vi "RLmodel GNSS-NtripClient.vi"() -> ()   [LabVIEW 2019]
uses:
  C:/Users/WEGO/Documents/GitHub/Ycar/LabVIEW/Gmap/dll/GMap.NET.WindowsForms.dll
  Gmap/dll/GMap.NET.WindowsForms.dll
  Ctrl/ublox-ui_main.ctl
  Ctrl/gnss_config-2.ctl
  Ctrl/Ntrip_Account_db.ctl
  Ctrl/cmd_common.ctl
  Ctrl/cmd_ini-add-read.ctl
  Ctrl/cmd_ini-RW.ctl
  Ctrl/GNSS-Ntrip ref.ctl
  Gmap/gmap_fgv-cmd.ctl
panel:
  out "GNSS time":string
  out "Ntrip conn":bool
  out "NMEA val":bool
  in  "main tap":T1(tab)
  in  "Send-Serial Start-Stop":bool
  in  "GNSS Start-Stop":bool
  out "TM\nptn":u32(slide) scale=0.0..200.0
  in  "GMapControl":refnum<k24>(container)
  out "Sea Level":dbl
  out "N of Satellites":i32
  out "TM graph":T2(graph)=[{"TM array"=[{"Y(E)"=195478.83340938148, "X(N)"=532749.6315443226}, {"Y(E)"=195478.83340938148, "X(N)"=532749.6315443226}, {"Y(E)"=195478.83340938148, "X(N)"=532749.6315443226}, {"Y(E)"=195478.83340938148, "X(N)"=532749.6315443226}, {"Y(E)"=195478.83340938148, "X(N)"=532749.6315443226}, {"Y(E)"=195478.83340938148, "X(N)"=532749.6315443226}, {"Y(E)"=195478.83340938148, "X(N)"=532749.6315443226}, {"Y(E)"=195478.83340938148, "X(N)"=532749.6315443226}, {"Y(E)"=195478.83340938148, "X(N)"=532749.6315443226}, {"Y(E)"=195478.83340938148, "X(N)"=532749.6315443226}, {"Y(E)"=195478.80387262133, "X(N)"=532749.5945652778}, {"Y(E)"=195478.80387262133, "X(N)"=532749.5945652778}, {"Y(E)"=195478.80387262133, "X(N)"=532749.5945652778}, {"Y(E)"=195478.80387262133, "X(N)"=532749.5945652778}, {"Y(E)"=195478.80387262133, "X(N)"=532749.5945652778}, {"Y(E)"=195478.80387262133, "X(N)"=532749.5945652778}, {"Y(E)"=195478.80387262133, "X(N)"=532749.5945652778}, {"Y(E)"=195478.80387262133, "X(N)"=532749.5945652778}, {"Y(E)"=195478.80387262133, "X(N)"=532749.5945652778}, {"Y(E)"=195478.80387262133, "X(N)"=532749.5945652778}, {"Y(E)"=195478.80387262133, "X(N)"=532749.5945652778}, {"Y(E)"=195478.80387262133, "X(N)"=532749.5945652778}, {"Y(E)"=195478.80387262133, "X(N)"=532749.5945652778}, {"Y(E)"=195478.86283602339, "X(N)"=532749.4650507653}, {"Y(E)"=195478.86283602339, "X(N)"=532749.4650507653}, {"Y(E)"=195478.86283602339, "X(N)"=532749.4650507653}, {"Y(E)"=195478.86283602339, "X(N)"=532749.4650507653}, {"Y(E)"=195478.86283602339, "X(N)"=532749.4650507653}, {"Y(E)"=195478.86283602339, "X(N)"=532749.4650507653}, {"Y(E)"=195478.86283602339, "X(N)"=532749.4650507653}, {"Y(E)"=195478.86283602339, "X(N)"=532749.4650507653}, {"Y(E)"=195478.86283602339, "X(N)"=532749.4650507653}, {"Y(E)"=195478.86283602339, "X(N)"=532749.4650507653}, {"Y(E)"=195478.86283602339, "X(N)"=532749.4650507653}, {"Y(E)"=195478.86283602339, "X(N)"=532749.4650507653}, {"Y(E)"=195478.86283602339, "X(N)"=532749.4650507653}, {"Y(E)"=195478.8185809412, "X(N)"=532749.5020697443}, {"Y(E)"=195478.8185809412, "X(N)"=532749.5020697443}, {"Y(E)"=195478.8185809412, "X(N)"=532749.5020697443}, {"Y(E)"=195478.8185809412, "X(N)"=532749.5020697443}, {"Y(E)"=195478.8185809412, "X(N)"=532749.5020697443}, {"Y(E)"=195478.8185809412, "X(N)"=532749.5020697443}, {"Y(E)"=195478.8185809412, "X(N)"=532749.5020697443}, {"Y(E)"=195478.8185809412, "X(N)"=532749.5020697443}, {"Y(E)"=195478.8185809412, "X(N)"=532749.5020697443}, {"Y(E)"=195478.8185809412, "X(N)"=532749.5020697443}, {"Y(E)"=195478.8185809412, "X(N)"=532749.5020697443}, {"Y(E)"=195478.8185809412, "X(N)"=532749.5020697443}, {"Y(E)"=195478.8185809412, "X(N)"=532749.5020697443}, {"Y(E)"=195478.8333493192, "X(N)"=532749.5205592669}, {"Y(E)"=195478.8333493192, "X(N)"=532749.5205592669}, {"Y(E)"=195478.8333493192, "X(N)"=532749.5205592669}, {"Y(E)"=195478.8333493192, "X(N)"=532749.5205592669}, {"Y(E)"=195478.8333493192, "X(N)"=532749.5205592669}, {"Y(E)"=195478.8333493192, "X(N)"=532749.5205592669}, {"Y(E)"=195478.8333493192, "X(N)"=532749.5205592669}, {"Y(E)"=195478.8333493192, "X(N)"=532749.5205592669}, {"Y(E)"=195478.8333493192, "X(N)"=532749.5205592669}, {"Y(E)"=195478.8333493192, "X(N)"=532749.5205592669}, {"Y(E)"=195478.8333493192, "X(N)"=532749.5205592669}, {"Y(E)"=195478.8333493192, "X(N)"=532749.5205592669}, {"Y(E)"=195478.81854089958, "X(N)"=532749.4280797082}, {"Y(E)"=195478.81854089958, "X(N)"=532749.4280797082}, {"Y(E)"=195478.81854089958, "X(N)"=532749.4280797082}, {"Y(E)"=195478.81854089958, "X(N)"=532749.4280797082}, {"Y(E)"=195478.81854089958, "X(N)"=532749.4280797082}, {"Y(E)"=195478.81854089958, "X(N)"=532749.4280797082}, {"Y(E)"=195478.81854089958, "X(N)"=532749.4280797082}, {"Y(E)"=195478.81854089958, "X(N)"=532749.4280797082}, {"Y(E)"=195478.81854089958, "X(N)"=532749.4280797082}, {"Y(E)"=195478.81854089958, "X(N)"=532749.4280797082}, {"Y(E)"=195478.81854089958, "X(N)"=532749.4280797082}, {"Y(E)"=195478.81854089958, "X(N)"=532749.4280797082}, {"Y(E)"=195478.81854089958, "X(N)"=532749.4280797082}, {"Y(E)"=195478.8332592258, "X(N)"=532749.3540816847}, {"Y(E)"=195478.8332592258, "X(N)"=532749.3540816847}, {"Y(E)"=195478.8332592258, "X(N)"=532749.3540816847}, {"Y(E)"=195478.8332592258, "X(N)"=532749.3540816847}, {"Y(E)"=195478.8332592258, "X(N)"=532749.3540816847}, {"Y(E)"=195478.8332592258, "X(N)"=532749.3540816847}, {"Y(E)"=195478.8332592258, "X(N)"=532749.3540816847}, {"Y(E)"=195478.8332592258, "X(N)"=532749.3540816847}, {"Y(E)"=195478.8332592258, "X(N)"=532749.3540816847}, {"Y(E)"=195478.8332592258, "X(N)"=532749.3540816847}, {"Y(E)"=195478.8332592258, "X(N)"=532749.3540816847}, {"Y(E)"=195478.8332592258, "X(N)"=532749.3540816847}, {"Y(E)"=195478.8332592258, "X(N)"=532749.3540816847}, {"Y(E)"=195478.61200383154, "X(N)"=532749.5761715989}, {"Y(E)"=195478.61200383154, "X(N)"=532749.5761715989}, {"Y(E)"=195478.61200383154, "X(N)"=532749.5761715989}, {"Y(E)"=195478.61200383154, "X(N)"=532749.5761715989}, {"Y(E)"=195478.61200383154, "X(N)"=532749.5761715989}, {"Y(E)"=195478.61200383154, "X(N)"=532749.5761715989}, {"Y(E)"=195478.61200383154, "X(N)"=532749.5761715989}, {"Y(E)"=195478.61200383154, "X(N)"=532749.5761715989}, {"Y(E)"=195478.61200383154, "X(N)"=532749.5761715989}, {"Y(E)"=195478.61200383154, "X(N)"=532749.5761715989}, {"Y(E)"=195478.61200383154, "X(N)"=532749.5761715989}, {"Y(E)"=195478.61200383154, "X(N)"=532749.5761715989}, {"Y(E)"=195478.61200383154, "X(N)"=532749.5761715989}, {"Y(E)"=195478.61197379892, "X(N)"=532749.5206790727}, {"Y(E)"=195478.61197379892, "X(N)"=532749.5206790727}, {"Y(E)"=195478.61197379892, "X(N)"=532749.5206790727}, {"Y(E)"=195478.61197379892, "X(N)"=532749.5206790727}, {"Y(E)"=195478.61197379892, "X(N)"=532749.5206790727}, {"Y(E)"=195478.61197379892, "X(N)"=532749.5206790727}, {"Y(E)"=195478.61197379892, "X(N)"=532749.5206790727}, {"Y(E)"=195478.61197379892, "X(N)"=532749.5206790727}, {"Y(E)"=195478.61197379892, "X(N)"=532749.5206790727}, {"Y(E)"=195478.61197379892, "X(N)"=532749.5206790727}, {"Y(E)"=195478.61197379892, "X(N)"=532749.5206790727}, {"Y(E)"=195478.61197379892, "X(N)"=532749.5206790727}, {"Y(E)"=195478.61197379892, "X(N)"=532749.5206790727}, {"Y(E)"=195478.64144048005, "X(N)"=532749.4281755526}, {"Y(E)"=195478.64144048005, "X(N)"=532749.4281755526}, {"Y(E)"=195478.64144048005, "X(N)"=532749.4281755526}, {"Y(E)"=195478.64144048005, "X(N)"=532749.4281755526}, {"Y(E)"=195478.64144048005, "X(N)"=532749.4281755526}, {"Y(E)"=195478.64144048005, "X(N)"=532749.4281755526}, {"Y(E)"=195478.64144048005, "X(N)"=532749.4281755526}, {"Y(E)"=195478.64144048005, "X(N)"=532749.4281755526}, {"Y(E)"=195478.64144048005, "X(N)"=532749.4281755526}, {"Y(E)"=195478.64144048005, "X(N)"=532749.4281755526}, {"Y(E)"=195478.64144048005, "X(N)"=532749.4281755526}, {"Y(E)"=195478.64144048005, "X(N)"=532749.4281755526}, {"Y(E)"=195478.64144048005, "X(N)"=532749.4281755526}, {"Y(E)"=195478.56754852948, "X(N)"=532749.2432403986}, {"Y(E)"=195478.56754852948, "X(N)"=532749.2432403986}, {"Y(E)"=195478.56754852948, "X(N)"=532749.2432403986}, {"Y(E)"=195478.56754852948, "X(N)"=532749.2432403986}, {"Y(E)"=195478.56754852948, "X(N)"=532749.2432403986}, {"Y(E)"=195478.56754852948, "X(N)"=532749.2432403986}, {"Y(E)"=195478.56754852948, "X(N)"=532749.2432403986}, {"Y(E)"=195478.56754852948, "X(N)"=532749.2432403986}, {"Y(E)"=195478.56754852948, "X(N)"=532749.2432403986}, {"Y(E)"=195478.56754852948, "X(N)"=532749.2432403986}, {"Y(E)"=195478.56754852948, "X(N)"=532749.2432403986}, {"Y(E)"=195478.56754852948, "X(N)"=532749.2432403986}, {"Y(E)"=195478.56754852948, "X(N)"=532749.2432403986}, {"Y(E)"=195478.5822568451, "X(N)"=532749.1507448669}, {"Y(E)"=195478.5822568451, "X(N)"=532749.1507448669}, {"Y(E)"=195478.5822568451, "X(N)"=532749.1507448669}, {"Y(E)"=195478.5822568451, "X(N)"=532749.1507448669}, {"Y(E)"=195478.5822568451, "X(N)"=532749.1507448669}, {"Y(E)"=195478.5822568451, "X(N)"=532749.1507448669}, {"Y(E)"=195478.5822568451, "X(N)"=532749.1507448669}, {"Y(E)"=195478.5822568451, "X(N)"=532749.1507448669}, {"Y(E)"=195478.5822568451, "X(N)"=532749.1507448669}, {"Y(E)"=195478.5822568451, "X(N)"=532749.1507448669}, {"Y(E)"=195478.5822568451, "X(N)"=532749.1507448669}, {"Y(E)"=195478.5822568451, "X(N)"=532749.1507448669}, {"Y(E)"=195478.5822568451, "X(N)"=532749.1507448669}, {"Y(E)"=195478.3755095352, "X(N)"=532748.9103890732}, {"Y(E)"=195478.3755095352, "X(N)"=532748.9103890732}, {"Y(E)"=195478.3755095352, "X(N)"=532748.9103890732}, {"Y(E)"=195478.3755095352, "X(N)"=532748.9103890732}, {"Y(E)"=195478.3755095352, "X(N)"=532748.9103890732}, {"Y(E)"=195478.3755095352, "X(N)"=532748.9103890732}, {"Y(E)"=195478.3755095352, "X(N)"=532748.9103890732}, {"Y(E)"=195478.3755095352, "X(N)"=532748.9103890732}, {"Y(E)"=195478.3755095352, "X(N)"=532748.9103890732}, {"Y(E)"=195478.3755095352, "X(N)"=532748.9103890732}, {"Y(E)"=195478.3755095352, "X(N)"=532748.9103890732}, {"Y(E)"=195478.3755095352, "X(N)"=532748.9103890732}, {"Y(E)"=195478.3755095352, "X(N)"=532748.9103890732}, {"Y(E)"=195478.37543945547, "X(N)"=532748.78090651}, {"Y(E)"=195478.37543945547, "X(N)"=532748.78090651}, {"Y(E)"=195478.37543945547, "X(N)"=532748.78090651}, {"Y(E)"=195478.37543945547, "X(N)"=532748.78090651}, {"Y(E)"=195478.37543945547, "X(N)"=532748.78090651}, {"Y(E)"=195478.37543945547, "X(N)"=532748.78090651}, {"Y(E)"=195478.37543945547, "X(N)"=532748.78090651}, {"Y(E)"=195478.37543945547, "X(N)"=532748.78090651}, {"Y(E)"=195478.37543945547, "X(N)"=532748.78090651}, {"Y(E)"=195478.37543945547, "X(N)"=532748.78090651}, {"Y(E)"=195478.37543945547, "X(N)"=532748.78090651}, {"Y(E)"=195478.37543945547, "X(N)"=532748.78090651}, {"Y(E)"=195478.5082848043, "X(N)"=532748.8178296402}, {"Y(E)"=195478.5082848043, "X(N)"=532748.8178296402}, {"Y(E)"=195478.5082848043, "X(N)"=532748.8178296402}, {"Y(E)"=195478.5082848043, "X(N)"=532748.8178296402}, {"Y(E)"=195478.5082848043, "X(N)"=532748.8178296402}, {"Y(E)"=195478.5082848043, "X(N)"=532748.8178296402}, {"Y(E)"=195478.5082848043, "X(N)"=532748.8178296402}, {"Y(E)"=195478.5082848043, "X(N)"=532748.8178296402}, {"Y(E)"=195478.5082848043, "X(N)"=532748.8178296402}, {"Y(E)"=195478.5082848043, "X(N)"=532748.8178296402}, {"Y(E)"=195478.5082848043, "X(N)"=532748.8178296402}, {"Y(E)"=195478.5082848043, "X(N)"=532748.8178296402}, {"Y(E)"=195478.5082848043, "X(N)"=532748.8178296402}, {"Y(E)"=195478.7001636224, "X(N)"=532748.8547208244}, {"Y(E)"=195478.7001636224, "X(N)"=532748.8547208244}, {"Y(E)"=195478.7001636224, "X(N)"=532748.8547208244}, {"Y(E)"=195478.7001636224, "X(N)"=532748.8547208244}, {"Y(E)"=195478.7001636224, "X(N)"=532748.8547208244}, {"Y(E)"=195478.7001636224, "X(N)"=532748.8547208244}, {"Y(E)"=195478.7001636224, "X(N)"=532748.8547208244}, {"Y(E)"=195478.7001636224, "X(N)"=532748.8547208244}, {"Y(E)"=195478.7001636224, "X(N)"=532748.8547208244}, {"Y(E)"=195478.7001636224, "X(N)"=532748.8547208244}]}, {"TM array"=[{"Y(E)"=195478.60442441847, "X(N)"=532749.6892681528}, {"Y(E)"=195478.63475492285, "X(N)"=532749.6883149784}, {"Y(E)"=195478.6649657266, "X(N)"=532749.6854592166}, {"Y(E)"=195478.69493760145, "X(N)"=532749.680712138}, {"Y(E)"=195478.72455226214, "X(N)"=532749.6740924771}, {"Y(E)"=195478.7536928331, "X(N)"=532749.6656263586}, {"Y(E)"=195478.7822443098, "X(N)"=532749.6553471944}, {"Y(E)"=195478.81009401265, "X(N)"=532749.6432955518}, {"Y(E)"=195478.83713203156, "X(N)"=532749.6295189931}, {"Y(E)"=195478.86325165984, "X(N)"=532749.6140718879}, {"Y(E)"=195478.88834981524, "X(N)"=532749.5970151991}, {"Y(E)"=195478.91232744683, "X(N)"=532749.5784162417}, {"Y(E)"=195478.93508992583, "X(N)"=532749.5583484169}, {"Y(E)"=195478.95654741913, "X(N)"=532749.5368909236}, {"Y(E)"=195478.97661524382, "X(N)"=532749.5141284446}, {"Y(E)"=195478.99521420136, "X(N)"=532749.490150813}, {"Y(E)"=195479.01227089018, "X(N)"=532749.4650526576}, {"Y(E)"=195479.02771799528, "X(N)"=532749.4389330294}, {"Y(E)"=195479.04149455403, "X(N)"=532749.4118950105}, {"Y(E)"=195479.0535461966, "X(N)"=532749.3840453076}, {"Y(E)"=195479.06382536073, "X(N)"=532749.3554938309}, {"Y(E)"=195479.0722914792, "X(N)"=532749.32635326}, {"Y(E)"=195479.07891114015, "X(N)"=532749.2967385993}, {"Y(E)"=195479.0836582188, "X(N)"=532749.2667667244}, {"Y(E)"=195479.08651398055, "X(N)"=532749.2365559207}, {"Y(E)"=195479.08746715504, "X(N)"=532749.2062254163}, {"Y(E)"=195479.08651398055, "X(N)"=532749.1758949119}, {"Y(E)"=195479.0836582188, "X(N)"=532749.1456841081}, {"Y(E)"=195479.07891114015, "X(N)"=532749.1157122332}, {"Y(E)"=195479.0722914792, "X(N)"=532749.0860975726}, {"Y(E)"=195479.06382536073, "X(N)"=532749.0569570017}, {"Y(E)"=195479.0535461966, "X(N)"=532749.0284055249}, {"Y(E)"=195479.04149455403, "X(N)"=532749.000555822}, {"Y(E)"=195479.02771799528, "X(N)"=532748.9735178031}, {"Y(E)"=195479.01227089018, "X(N)"=532748.9473981749}, {"Y(E)"=195478.99521420136, "X(N)"=532748.9223000195}, {"Y(E)"=195478.97661524382, "X(N)"=532748.898322388}, {"Y(E)"=195478.95654741913, "X(N)"=532748.8755599089}, {"Y(E)"=195478.93508992583, "X(N)"=532748.8541024156}, {"Y(E)"=195478.91232744683, "X(N)"=532748.8340345909}, {"Y(E)"=195478.88834981524, "X(N)"=532748.8154356334}, {"Y(E)"=195478.86325165984, "X(N)"=532748.7983789446}, {"Y(E)"=195478.83713203156, "X(N)"=532748.7829318395}, {"Y(E)"=195478.81009401265, "X(N)"=532748.7691552808}, {"Y(E)"=195478.7822443098, "X(N)"=532748.7571036381}, {"Y(E)"=195478.7536928331, "X(N)"=532748.746824474}, {"Y(E)"=195478.72455226214, "X(N)"=532748.7383583555}, {"Y(E)"=195478.69493760145, "X(N)"=532748.7317386946}, {"Y(E)"=195478.6649657266, "X(N)"=532748.726991616}, {"Y(E)"=195478.63475492285, "X(N)"=532748.7241358542}, {"Y(E)"=195478.60442441847, "X(N)"=532748.7231826797}, {"Y(E)"=195478.5740939141, "X(N)"=532748.7241358542}, {"Y(E)"=195478.54388311034, "X(N)"=532748.726991616}, {"Y(E)"=195478.5139112355, "X(N)"=532748.7317386946}, {"Y(E)"=195478.4842965748, "X(N)"=532748.7383583555}, {"Y(E)"=195478.45515600385, "X(N)"=532748.746824474}, {"Y(E)"=195478.42660452714, "X(N)"=532748.7571036381}, {"Y(E)"=195478.3987548243, "X(N)"=532748.7691552808}, {"Y(E)"=195478.37171680538, "X(N)"=532748.7829318395}, {"Y(E)"=195478.3455971771, "X(N)"=532748.7983789446}, {"Y(E)"=195478.3204990217, "X(N)"=532748.8154356334}, {"Y(E)"=195478.29652139012, "X(N)"=532748.8340345909}, {"Y(E)"=195478.27375891112, "X(N)"=532748.8541024156}, {"Y(E)"=195478.25230141782, "X(N)"=532748.8755599089}, {"Y(E)"=195478.23223359312, "X(N)"=532748.898322388}, {"Y(E)"=195478.21363463558, "X(N)"=532748.9223000195}, {"Y(E)"=195478.19657794677, "X(N)"=532748.9473981749}, {"Y(E)"=195478.18113084167, "X(N)"=532748.9735178031}, {"Y(E)"=195478.16735428292, "X(N)"=532749.000555822}, {"Y(E)"=195478.15530264034, "X(N)"=532749.0284055249}, {"Y(E)"=195478.14502347622, "X(N)"=532749.0569570017}, {"Y(E)"=195478.13655735774, "X(N)"=532749.0860975726}, {"Y(E)"=195478.1299376968, "X(N)"=532749.1157122332}, {"Y(E)"=195478.12519061816, "X(N)"=532749.1456841081}, {"Y(E)"=195478.1223348564, "X(N)"=532749.1758949119}, {"Y(E)"=195478.1213816819, "X(N)"=532749.2062254163}, {"Y(E)"=195478.1223348564, "X(N)"=532749.2365559207}, {"Y(E)"=195478.12519061816, "X(N)"=532749.2667667244}, {"Y(E)"=195478.1299376968, "X(N)"=532749.2967385993}, {"Y(E)"=195478.13655735774, "X(N)"=532749.32635326}, {"Y(E)"=195478.14502347622, "X(N)"=532749.3554938309}, {"Y(E)"=195478.15530264034, "X(N)"=532749.3840453076}, {"Y(E)"=195478.16735428292, "X(N)"=532749.4118950105}, {"Y(E)"=195478.18113084167, "X(N)"=532749.4389330294}, {"Y(E)"=195478.19657794677, "X(N)"=532749.4650526576}, {"Y(E)"=195478.21363463558, "X(N)"=532749.490150813}, {"Y(E)"=195478.23223359312, "X(N)"=532749.5141284446}, {"Y(E)"=195478.25230141782, "X(N)"=532749.5368909236}, {"Y(E)"=195478.27375891112, "X(N)"=532749.5583484169}, {"Y(E)"=195478.29652139012, "X(N)"=532749.5784162417}, {"Y(E)"=195478.3204990217, "X(N)"=532749.5970151991}, {"Y(E)"=195478.3455971771, "X(N)"=532749.6140718879}, {"Y(E)"=195478.37171680538, "X(N)"=532749.6295189931}, {"Y(E)"=195478.3987548243, "X(N)"=532749.6432955518}, {"Y(E)"=195478.42660452714, "X(N)"=532749.6553471944}, {"Y(E)"=195478.45515600385, "X(N)"=532749.6656263586}, {"Y(E)"=195478.4842965748, "X(N)"=532749.6740924771}, {"Y(E)"=195478.5139112355, "X(N)"=532749.680712138}, {"Y(E)"=195478.54388311034, "X(N)"=532749.6854592166}, {"Y(E)"=195478.5740939141, "X(N)"=532749.6883149784}, {"Y(E)"=195478.60442441847, "X(N)"=532749.6892681528}]}, {"TM array"=[{"Y(E)"=195478.60442441847, "X(N)"=532750.2062254163}, {"Y(E)"=195478.667214938, "X(N)"=532750.2042521447}, {"Y(E)"=195478.72975765204, "X(N)"=532750.1983401176}, {"Y(E)"=195478.79180573305, "X(N)"=532750.188512667}, {"Y(E)"=195478.85311430565, "X(N)"=532750.1748085774}, {"Y(E)"=195478.91344141285, "X(N)"=532750.1572819325}, {"Y(E)"=195478.97254897116, "X(N)"=532750.1360019022}, {"Y(E)"=195479.03020371005, "X(N)"=532750.1110524688}, {"Y(E)"=195479.08617809258, "X(N)"=532750.0825320963}, {"Y(E)"=195479.14025121345, "X(N)"=532750.0505533417}, {"Y(E)"=195479.19220967076, "X(N)"=532750.0152424106}, {"Y(E)"=195479.24184840822, "X(N)"=532749.9767386591}, {"Y(E)"=195479.2889715244, "X(N)"=532749.9351940437}, {"Y(E)"=195479.3333930459, "X(N)"=532749.8907725222}, {"Y(E)"=195479.37493766125, "X(N)"=532749.843649406}, {"Y(E)"=195479.41344141285, "X(N)"=532749.7940106685}, {"Y(E)"=195479.44875234397, "X(N)"=532749.7420522113}, {"Y(E)"=195479.4807310985, "X(N)"=532749.6879790904}, {"Y(E)"=195479.50925147094, "X(N)"=532749.6320047078}, {"Y(E)"=195479.53420090437, "X(N)"=532749.5743499689}, {"Y(E)"=195479.55548093477, "X(N)"=532749.5152424106}, {"Y(E)"=195479.5730075796, "X(N)"=532749.4549153034}, {"Y(E)"=195479.5867116692, "X(N)"=532749.3936067309}, {"Y(E)"=195479.59653911978, "X(N)"=532749.3315586499}, {"Y(E)"=195479.6024511469, "X(N)"=532749.2690159358}, {"Y(E)"=195479.60442441847, "X(N)"=532749.2062254163}, {"Y(E)"=195479.6024511469, "X(N)"=532749.1434348967}, {"Y(E)"=195479.59653911978, "X(N)"=532749.0808921827}, {"Y(E)"=195479.5867116692, "X(N)"=532749.0188441017}, {"Y(E)"=195479.5730075796, "X(N)"=532748.9575355292}, {"Y(E)"=195479.55548093477, "X(N)"=532748.897208422}, {"Y(E)"=195479.53420090437, "X(N)"=532748.8381008636}, {"Y(E)"=195479.50925147094, "X(N)"=532748.7804461247}, {"Y(E)"=195479.4807310985, "X(N)"=532748.7244717422}, {"Y(E)"=195479.44875234397, "X(N)"=532748.6703986212}, {"Y(E)"=195479.41344141285, "X(N)"=532748.618440164}, {"Y(E)"=195479.37493766125, "X(N)"=532748.5688014266}, {"Y(E)"=195479.3333930459, "X(N)"=532748.5216783104}, {"Y(E)"=195479.2889715244, "X(N)"=532748.4772567889}, {"Y(E)"=195479.24184840822, "X(N)"=532748.4357121735}, {"Y(E)"=195479.19220967076, "X(N)"=532748.397208422}, {"Y(E)"=195479.14025121345, "X(N)"=532748.3618974908}, {"Y(E)"=195479.08617809258, "X(N)"=532748.3299187362}, {"Y(E)"=195479.03020371005, "X(N)"=532748.3013983638}, {"Y(E)"=195478.97254897116, "X(N)"=532748.2764489304}, {"Y(E)"=195478.91344141285, "X(N)"=532748.2551689}, {"Y(E)"=195478.85311430565, "X(N)"=532748.2376422551}, {"Y(E)"=195478.79180573305, "X(N)"=532748.2239381656}, {"Y(E)"=195478.72975765204, "X(N)"=532748.214110715}, {"Y(E)"=195478.667214938, "X(N)"=532748.2081986879}, {"Y(E)"=195478.60442441847, "X(N)"=532748.2062254163}, {"Y(E)"=195478.54163389895, "X(N)"=532748.2081986879}, {"Y(E)"=195478.4790911849, "X(N)"=532748.214110715}, {"Y(E)"=195478.4170431039, "X(N)"=532748.2239381656}, {"Y(E)"=195478.3557345313, "X(N)"=532748.2376422551}, {"Y(E)"=195478.2954074241, "X(N)"=532748.2551689}, {"Y(E)"=195478.2362998658, "X(N)"=532748.2764489304}, {"Y(E)"=195478.1786451269, "X(N)"=532748.3013983638}, {"Y(E)"=195478.12267074437, "X(N)"=532748.3299187362}, {"Y(E)"=195478.0685976235, "X(N)"=532748.3618974908}, {"Y(E)"=195478.0166391662, "X(N)"=532748.397208422}, {"Y(E)"=195477.96700042873, "X(N)"=532748.4357121735}, {"Y(E)"=195477.91987731255, "X(N)"=532748.4772567889}, {"Y(E)"=195477.87545579104, "X(N)"=532748.5216783104}, {"Y(E)"=195477.8339111757, "X(N)"=532748.5688014266}, {"Y(E)"=195477.7954074241, "X(N)"=532748.618440164}, {"Y(E)"=195477.76009649297, "X(N)"=532748.6703986212}, {"Y(E)"=195477.72811773844, "X(N)"=532748.7244717422}, {"Y(E)"=195477.699597366, "X(N)"=532748.7804461247}, {"Y(E)"=195477.67464793258, "X(N)"=532748.8381008636}, {"Y(E)"=195477.65336790218, "X(N)"=532748.897208422}, {"Y(E)"=195477.63584125735, "X(N)"=532748.9575355292}, {"Y(E)"=195477.62213716775, "X(N)"=532749.0188441017}, {"Y(E)"=195477.61230971717, "X(N)"=532749.0808921827}, {"Y(E)"=195477.60639769005, "X(N)"=532749.1434348967}, {"Y(E)"=195477.60442441847, "X(N)"=532749.2062254163}, {"Y(E)"=195477.60639769005, "X(N)"=532749.2690159358}, {"Y(E)"=195477.61230971717, "X(N)"=532749.3315586499}, {"Y(E)"=195477.62213716775, "X(N)"=532749.3936067309}, {"Y(E)"=195477.63584125735, "X(N)"=532749.4549153034}, {"Y(E)"=195477.65336790218, "X(N)"=532749.5152424106}, {"Y(E)"=195477.67464793258, "X(N)"=532749.5743499689}, {"Y(E)"=195477.699597366, "X(N)"=532749.6320047078}, {"Y(E)"=195477.72811773844, "X(N)"=532749.6879790904}, {"Y(E)"=195477.76009649297, "X(N)"=532749.7420522113}, {"Y(E)"=195477.7954074241, "X(N)"=532749.7940106685}, {"Y(E)"=195477.8339111757, "X(N)"=532749.843649406}, {"Y(E)"=195477.87545579104, "X(N)"=532749.8907725222}, {"Y(E)"=195477.91987731255, "X(N)"=532749.9351940437}, {"Y(E)"=195477.96700042873, "X(N)"=532749.9767386591}, {"Y(E)"=195478.0166391662, "X(N)"=532750.0152424106}, {"Y(E)"=195478.0685976235, "X(N)"=532750.0505533417}, {"Y(E)"=195478.12267074437, "X(N)"=532750.0825320963}, {"Y(E)"=195478.1786451269, "X(N)"=532750.1110524688}, {"Y(E)"=195478.2362998658, "X(N)"=532750.1360019022}, {"Y(E)"=195478.2954074241, "X(N)"=532750.1572819325}, {"Y(E)"=195478.3557345313, "X(N)"=532750.1748085774}, {"Y(E)"=195478.4170431039, "X(N)"=532750.188512667}, {"Y(E)"=195478.4790911849, "X(N)"=532750.1983401176}, {"Y(E)"=195478.54163389895, "X(N)"=532750.2042521447}, {"Y(E)"=195478.60442441847, "X(N)"=532750.2062254163}]}, {"TM array"=[{"Y(E)"=195478.60442441847, "X(N)"=532751.2062254163}, {"Y(E)"=195478.73000545753, "X(N)"=532751.2022788732}, {"Y(E)"=195478.8550908856, "X(N)"=532751.1904548189}, {"Y(E)"=195478.97918704763, "X(N)"=532751.1707999178}, {"Y(E)"=195479.10180419282, "X(N)"=532751.1433917385}, {"Y(E)"=195479.22245840722, "X(N)"=532751.1083384489}, {"Y(E)"=195479.34067352384, "X(N)"=532751.0657783881}, {"Y(E)"=195479.4559830016, "X(N)"=532751.0158795213}, {"Y(E)"=195479.56793176668, "X(N)"=532750.9588387763}, {"Y(E)"=195479.67607800843, "X(N)"=532750.8948812673}, {"Y(E)"=195479.77999492307, "X(N)"=532750.824259405}, {"Y(E)"=195479.879272398, "X(N)"=532750.7472519018}, {"Y(E)"=195479.97351863034, "X(N)"=532750.6641626711}, {"Y(E)"=195480.0623616733, "X(N)"=532750.5753196281}, {"Y(E)"=195480.14545090403, "X(N)"=532750.4810733958}, {"Y(E)"=195480.22245840722, "X(N)"=532750.3817959209}, {"Y(E)"=195480.29308026948, "X(N)"=532750.2778790062}, {"Y(E)"=195480.35703777857, "X(N)"=532750.1697327645}, {"Y(E)"=195480.4140785234, "X(N)"=532750.0577839994}, {"Y(E)"=195480.46397739026, "X(N)"=532749.9424745217}, {"Y(E)"=195480.50653745106, "X(N)"=532749.824259405}, {"Y(E)"=195480.54159074073, "X(N)"=532749.7036051906}, {"Y(E)"=195480.56899891995, "X(N)"=532749.5809880454}, {"Y(E)"=195480.5886538211, "X(N)"=532749.4568918834}, {"Y(E)"=195480.60047787533, "X(N)"=532749.3318064554}, {"Y(E)"=195480.60442441847, "X(N)"=532749.2062254163}, {"Y(E)"=195480.60047787533, "X(N)"=532749.0806443772}, {"Y(E)"=195480.5886538211, "X(N)"=532748.9555589492}, {"Y(E)"=195480.56899891995, "X(N)"=532748.8314627871}, {"Y(E)"=195480.54159074073, "X(N)"=532748.7088456419}, {"Y(E)"=195480.50653745106, "X(N)"=532748.5881914275}, {"Y(E)"=195480.46397739026, "X(N)"=532748.4699763109}, {"Y(E)"=195480.4140785234, "X(N)"=532748.3546668332}, {"Y(E)"=195480.35703777857, "X(N)"=532748.2427180681}, {"Y(E)"=195480.29308026948, "X(N)"=532748.1345718263}, {"Y(E)"=195480.22245840722, "X(N)"=532748.0306549117}, {"Y(E)"=195480.14545090403, "X(N)"=532747.9313774367}, {"Y(E)"=195480.0623616733, "X(N)"=532747.8371312044}, {"Y(E)"=195479.97351863034, "X(N)"=532747.7482881615}, {"Y(E)"=195479.879272398, "X(N)"=532747.6651989308}, {"Y(E)"=195479.77999492307, "X(N)"=532747.5881914275}, {"Y(E)"=195479.67607800843, "X(N)"=532747.5175695652}, {"Y(E)"=195479.56793176668, "X(N)"=532747.4536120562}, {"Y(E)"=195479.4559830016, "X(N)"=532747.3965713113}, {"Y(E)"=195479.34067352384, "X(N)"=532747.3466724445}, {"Y(E)"=195479.22245840722, "X(N)"=532747.3041123836}, {"Y(E)"=195479.10180419282, "X(N)"=532747.269059094}, {"Y(E)"=195478.97918704763, "X(N)"=532747.2416509148}, {"Y(E)"=195478.8550908856, "X(N)"=532747.2219960137}, {"Y(E)"=195478.73000545753, "X(N)"=532747.2101719594}, {"Y(E)"=195478.60442441847, "X(N)"=532747.2062254163}, {"Y(E)"=195478.47884337942, "X(N)"=532747.2101719594}, {"Y(E)"=195478.35375795135, "X(N)"=532747.2219960137}, {"Y(E)"=195478.22966178932, "X(N)"=532747.2416509148}, {"Y(E)"=195478.10704464413, "X(N)"=532747.269059094}, {"Y(E)"=195477.98639042972, "X(N)"=532747.3041123836}, {"Y(E)"=195477.8681753131, "X(N)"=532747.3466724445}, {"Y(E)"=195477.75286583535, "X(N)"=532747.3965713113}, {"Y(E)"=195477.64091707027, "X(N)"=532747.4536120562}, {"Y(E)"=195477.53277082852, "X(N)"=532747.5175695652}, {"Y(E)"=195477.42885391388, "X(N)"=532747.5881914275}, {"Y(E)"=195477.32957643896, "X(N)"=532747.6651989308}, {"Y(E)"=195477.2353302066, "X(N)"=532747.7482881615}, {"Y(E)"=195477.14648716364, "X(N)"=532747.8371312044}, {"Y(E)"=195477.0633979329, "X(N)"=532747.9313774367}, {"Y(E)"=195476.98639042972, "X(N)"=532748.0306549117}, {"Y(E)"=195476.91576856747, "X(N)"=532748.1345718263}, {"Y(E)"=195476.85181105838, "X(N)"=532748.2427180681}, {"Y(E)"=195476.79477031354, "X(N)"=532748.3546668332}, {"Y(E)"=195476.7448714467, "X(N)"=532748.4699763109}, {"Y(E)"=195476.7023113859, "X(N)"=532748.5881914275}, {"Y(E)"=195476.66725809622, "X(N)"=532748.7088456419}, {"Y(E)"=195476.639849917, "X(N)"=532748.8314627871}, {"Y(E)"=195476.62019501586, "X(N)"=532748.9555589492}, {"Y(E)"=195476.60837096162, "X(N)"=532749.0806443772}, {"Y(E)"=195476.60442441847, "X(N)"=532749.2062254163}, {"Y(E)"=195476.60837096162, "X(N)"=532749.3318064554}, {"Y(E)"=195476.62019501586, "X(N)"=532749.4568918834}, {"Y(E)"=195476.639849917, "X(N)"=532749.5809880454}, {"Y(E)"=195476.66725809622, "X(N)"=532749.7036051906}, {"Y(E)"=195476.7023113859, "X(N)"=532749.824259405}, {"Y(E)"=195476.7448714467, "X(N)"=532749.9424745217}, {"Y(E)"=195476.79477031354, "X(N)"=532750.0577839994}, {"Y(E)"=195476.85181105838, "X(N)"=532750.1697327645}, {"Y(E)"=195476.91576856747, "X(N)"=532750.2778790062}, {"Y(E)"=195476.98639042972, "X(N)"=532750.3817959209}, {"Y(E)"=195477.0633979329, "X(N)"=532750.4810733958}, {"Y(E)"=195477.14648716364, "X(N)"=532750.5753196281}, {"Y(E)"=195477.2353302066, "X(N)"=532750.6641626711}, {"Y(E)"=195477.32957643896, "X(N)"=532750.7472519018}, {"Y(E)"=195477.42885391388, "X(N)"=532750.824259405}, {"Y(E)"=195477.53277082852, "X(N)"=532750.8948812673}, {"Y(E)"=195477.64091707027, "X(N)"=532750.9588387763}, {"Y(E)"=195477.75286583535, "X(N)"=532751.0158795213}, {"Y(E)"=195477.8681753131, "X(N)"=532751.0657783881}, {"Y(E)"=195477.98639042972, "X(N)"=532751.1083384489}, {"Y(E)"=195478.10704464413, "X(N)"=532751.1433917385}, {"Y(E)"=195478.22966178932, "X(N)"=532751.1707999178}, {"Y(E)"=195478.35375795135, "X(N)"=532751.1904548189}, {"Y(E)"=195478.47884337942, "X(N)"=532751.2022788732}, {"Y(E)"=195478.60442441847, "X(N)"=532751.2062254163}]}, {"TM array"=[{"Y(E)"=195478.60442441847, "X(N)"=532752.2062254163}, {"Y(E)"=195478.79279597706, "X(N)"=532752.2003056016}, {"Y(E)"=195478.98042411916, "X(N)"=532752.1825695202}, {"Y(E)"=195479.16656836224, "X(N)"=532752.1530871685}, {"Y(E)"=195479.35049407996, "X(N)"=532752.1119748997}, {"Y(E)"=195479.5314754016, "X(N)"=532752.0593949652}, {"Y(E)"=195479.70879807652, "X(N)"=532751.995554874}, {"Y(E)"=195479.88176229317, "X(N)"=532751.9207065736}, {"Y(E)"=195480.04968544078, "X(N)"=532751.8351454564}, {"Y(E)"=195480.2119048034, "X(N)"=532751.7392091928}, {"Y(E)"=195480.36778017535, "X(N)"=532751.6332763993}, {"Y(E)"=195480.51669638773, "X(N)"=532751.5177651446}, {"Y(E)"=195480.65806573626, "X(N)"=532751.3931312986}, {"Y(E)"=195480.79133030074, "X(N)"=532751.259866734}, {"Y(E)"=195480.9159641468, "X(N)"=532751.1184973855}, {"Y(E)"=195481.0314754016, "X(N)"=532750.9695811732}, {"Y(E)"=195481.13740819498, "X(N)"=532750.8137058013}, {"Y(E)"=195481.2333444586, "X(N)"=532750.6514864386}, {"Y(E)"=195481.31890557587, "X(N)"=532750.483563291}, {"Y(E)"=195481.39375387615, "X(N)"=532750.3105990743}, {"Y(E)"=195481.45759396735, "X(N)"=532750.1332763993}, {"Y(E)"=195481.51017390186, "X(N)"=532749.9522950777}, {"Y(E)"=195481.55128617067, "X(N)"=532749.76836936}, {"Y(E)"=195481.58076852243, "X(N)"=532749.582225117}, {"Y(E)"=195481.59850460375, "X(N)"=532749.3945969748}, {"Y(E)"=195481.60442441847, "X(N)"=532749.2062254163}, {"Y(E)"=195481.59850460375, "X(N)"=532749.0178538577}, {"Y(E)"=195481.58076852243, "X(N)"=532748.8302257155}, {"Y(E)"=195481.55128617067, "X(N)"=532748.6440814725}, {"Y(E)"=195481.51017390186, "X(N)"=532748.4601557548}, {"Y(E)"=195481.45759396735, "X(N)"=532748.2791744332}, {"Y(E)"=195481.39375387615, "X(N)"=532748.1018517582}, {"Y(E)"=195481.31890557587, "X(N)"=532747.9288875415}, {"Y(E)"=195481.2333444586, "X(N)"=532747.760964394}, {"Y(E)"=195481.13740819498, "X(N)"=532747.5987450313}, {"Y(E)"=195481.0314754016, "X(N)"=532747.4428696594}, {"Y(E)"=195480.9159641468, "X(N)"=532747.293953447}, {"Y(E)"=195480.79133030074, "X(N)"=532747.1525840985}, {"Y(E)"=195480.65806573626, "X(N)"=532747.019319534}, {"Y(E)"=195480.51669638773, "X(N)"=532746.894685688}, {"Y(E)"=195480.36778017535, "X(N)"=532746.7791744332}, {"Y(E)"=195480.2119048034, "X(N)"=532746.6732416397}, {"Y(E)"=195480.04968544078, "X(N)"=532746.5773053762}, {"Y(E)"=195479.88176229317, "X(N)"=532746.4917442589}, {"Y(E)"=195479.70879807652, "X(N)"=532746.4168959586}, {"Y(E)"=195479.5314754016, "X(N)"=532746.3530558674}, {"Y(E)"=195479.35049407996, "X(N)"=532746.3004759329}, {"Y(E)"=195479.16656836224, "X(N)"=532746.2593636641}, {"Y(E)"=195478.98042411916, "X(N)"=532746.2298813123}, {"Y(E)"=195478.79279597706, "X(N)"=532746.212145231}, {"Y(E)"=195478.60442441847, "X(N)"=532746.2062254163}, {"Y(E)"=195478.4160528599, "X(N)"=532746.212145231}, {"Y(E)"=195478.2284247178, "X(N)"=532746.2298813123}, {"Y(E)"=195478.0422804747, "X(N)"=532746.2593636641}, {"Y(E)"=195477.858354757, "X(N)"=532746.3004759329}, {"Y(E)"=195477.67737343535, "X(N)"=532746.3530558674}, {"Y(E)"=195477.50005076043, "X(N)"=532746.4168959586}, {"Y(E)"=195477.32708654378, "X(N)"=532746.4917442589}, {"Y(E)"=195477.15916339617, "X(N)"=532746.5773053762}, {"Y(E)"=195476.99694403354, "X(N)"=532746.6732416397}, {"Y(E)"=195476.8410686616, "X(N)"=532746.7791744332}, {"Y(E)"=195476.69215244922, "X(N)"=532746.894685688}, {"Y(E)"=195476.55078310068, "X(N)"=532747.019319534}, {"Y(E)"=195476.4175185362, "X(N)"=532747.1525840985}, {"Y(E)"=195476.29288469013, "X(N)"=532747.293953447}, {"Y(E)"=195476.17737343535, "X(N)"=532747.4428696594}, {"Y(E)"=195476.07144064197, "X(N)"=532747.5987450313}, {"Y(E)"=195475.97550437835, "X(N)"=532747.760964394}, {"Y(E)"=195475.88994326108, "X(N)"=532747.9288875415}, {"Y(E)"=195475.8150949608, "X(N)"=532748.1018517582}, {"Y(E)"=195475.7512548696, "X(N)"=532748.2791744332}, {"Y(E)"=195475.6986749351, "X(N)"=532748.4601557548}, {"Y(E)"=195475.65756266628, "X(N)"=532748.6440814725}, {"Y(E)"=195475.62808031452, "X(N)"=532748.8302257155}, {"Y(E)"=195475.6103442332, "X(N)"=532749.0178538577}, {"Y(E)"=195475.60442441847, "X(N)"=532749.2062254163}, {"Y(E)"=195475.6103442332, "X(N)"=532749.3945969748}, {"Y(E)"=195475.62808031452, "X(N)"=532749.582225117}, {"Y(E)"=195475.65756266628, "X(N)"=532749.76836936}, {"Y(E)"=195475.6986749351, "X(N)"=532749.9522950777}, {"Y(E)"=195475.7512548696, "X(N)"=532750.1332763993}, {"Y(E)"=195475.8150949608, "X(N)"=532750.3105990743}, {"Y(E)"=195475.88994326108, "X(N)"=532750.483563291}, {"Y(E)"=195475.97550437835, "X(N)"=532750.6514864386}, {"Y(E)"=195476.07144064197, "X(N)"=532750.8137058013}, {"Y(E)"=195476.17737343535, "X(N)"=532750.9695811732}, {"Y(E)"=195476.29288469013, "X(N)"=532751.1184973855}, {"Y(E)"=195476.4175185362, "X(N)"=532751.259866734}, {"Y(E)"=195476.55078310068, "X(N)"=532751.3931312986}, {"Y(E)"=195476.69215244922, "X(N)"=532751.5177651446}, {"Y(E)"=195476.8410686616, "X(N)"=532751.6332763993}, {"Y(E)"=195476.99694403354, "X(N)"=532751.7392091928}, {"Y(E)"=195477.15916339617, "X(N)"=532751.8351454564}, {"Y(E)"=195477.32708654378, "X(N)"=532751.9207065736}, {"Y(E)"=195477.50005076043, "X(N)"=532751.995554874}, {"Y(E)"=195477.67737343535, "X(N)"=532752.0593949652}, {"Y(E)"=195477.858354757, "X(N)"=532752.1119748997}, {"Y(E)"=195478.0422804747, "X(N)"=532752.1530871685}, {"Y(E)"=195478.2284247178, "X(N)"=532752.1825695202}, {"Y(E)"=195478.4160528599, "X(N)"=532752.2003056016}, {"Y(E)"=195478.60442441847, "X(N)"=532752.2062254163}]}]
  in  "stop":bool
  in  "gmap center":bool
  out "GNSS data info":T3 {"HDOP" scale=0.0..10.0; "PDOP" scale=0.0..10.0; "2D Acc.m" scale=0.0..10.0; "Latitude" format="%.9f"; "Longitude" format="%.9f"; "3D Acc.m" scale=0.0..10.0}
  in  "Gmap Lon":dbl format="%.7f"
  in  "Gmap Lat":dbl format="%.7f"
  in  "gnss tm config":T4(tab)
  out "gnss mode cnt":u32[](array[numeric])
  out "Histogram Graph":cluster{i32[], dbl[]}(graph)
  in  "gnss mode check":bool
  out "Min circle R":dbl format="%.2g"
  out "Points size":i32
  out "loop count":i32
  in  "tm data reset":bool
  in  "TMarr-size limit":i32=200
  in  "Ref r size":dbl=1.0 format="%.2f"
  in  "Auto\ncenter":bool
  in  "PinDropMrkr":T5(ring)=enum."red_dot" caption="Pin Drop Marker"
  out "xcenter_TM":dbl
  out "ycenter_TM":dbl
  in  "Lat Dbclk":dbl format="%.11f"
  in  "Lon Dbclk":dbl format="%.11f"
  in  "Center \nupdate s":i32=10000
  in  "zoom":dbl(slide) scale=3.0..20.0
  out "NMEA cluster":T6
  out "Sel NMEA":string
  in  "Sel NMEA type":T7(ring)=enum."$GPGGA"
  in  "GNSS Serial cfg":T8={"Port"="COM10", "rate"=115200}
  in  "GNSS Serial delay":u32=20
  out "Raw NMEA":string
  out "Serial bufferN":u32(graph)
  in  "Local Time offset":u32=9
  in  "Send-Serial config":T9={"NMEA out port"="", "baud rate"=9600}
  in  "Data w sel":bool
  in  "Send Serial delay ms":u32=900
  out "log path":string
  out "TM array":cluster{"Y(E)":dbl, "X(N)":dbl}[](array[cluster])
  out "error out":errorcluster
  out "Mount point arr":string[](array[string])
  in  "Ntrip accounts DB index":u32(slide) scale=0.0..9.0
  in  "Ntrip accounts DB":T10[](array[typedef])
  in  "update mount point":bool
  in  "Select Mount points":u16(ring)
  out "RTCM recv":string
  in  "Ntrip connect":bool
  out "SourceTable recv-str":string
  in  "Current Ntrip account":T10={"address"="gnss.eseoul.go.kr", "port "=2101, "id"="seoul", "pwd"="seoul", "ref pt"="YONS-RTCM32-M5"}
  # "GNSS/GPS Test Program"
  # "Build ver:"
  # "Made by ybbaek https://github.com/yunbum"
  # "RLmodel GNSS NtripClient"
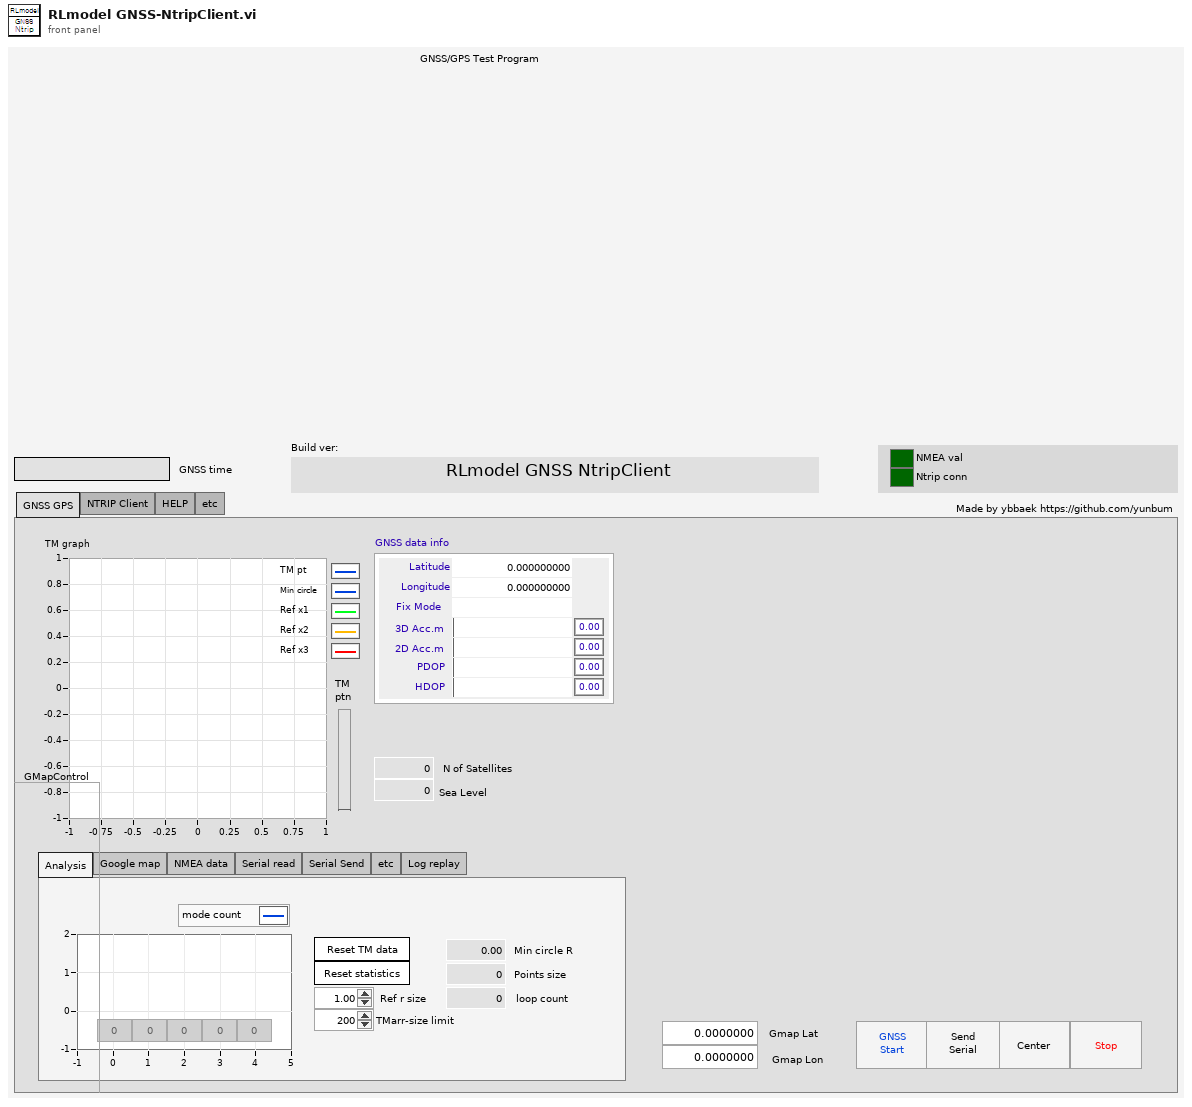
[diagram p1: front panel]
types:
  T1 = enum32{"GNSS GPS", "NTRIP Client", "HELP", "etc"}
  T2 = cluster{"TM array":cluster{"Y(E)":dbl, "X(N)":dbl}[]}[]
  T3 = typedef "ublox-ui_main.ctl" = cluster{"Latitude":dbl, "Longitude":dbl, "Fix Mode":string, "3D Acc.m":dbl, "2D Acc.m":dbl, "PDOP":dbl, "HDOP":dbl}
  T4 = enum32{"Analysis", "Google map", "NMEA data", "Serial read", "Serial Send", "etc", "Log replay"}
  T5 = enum16{"none", "arrow", "blue", "blue_small", "blue_dot", "blue_pushpin", "brown_small", "gray_small", "green", "green_small", "green_dot", "green_pushpin", "green_big_go", "yellow", "yellow_small", "yellow_dot", "yellow_big_pause", "yellow_pushpin", "lightblue", "lightblue_dot", "lightblue_pushpin", "orange", "orange_small", "orange_dot", "pink", "pink_dot", "pink_pushpin", "purple", "purple_small", "purple_dot", "purple_pushpin", "red", "red_small", "red_dot", "red_pushpin", "red_big_stop", "black_small", "white_small"}
  T6 = cluster{"GxGGA":string, "GxGSV":string, "GNRMC":string, "GxTXT":string, "GxGSA":string, "GxGLL":string}
  T7 = enum16{"$GPGSV", "$GLGSV", "$GPGGA", "$GAGSV", "$GBGSV", "$GNGLL", "$GNGGA", "$GNGSA", "$GNRMC", "$GNVTG"}
  T8 = typedef "gnss_config-2.ctl" = cluster{"Port":refnum<visa-resource-name>, "rate":u32}
  T9 = cluster{"NMEA out port":refnum<visa-resource-name>, "baud rate":u32}
  T10 = typedef "Ntrip_Account_db.ctl" = cluster{"address":string, "port ":u16, "id":string, "pwd":string, "ref pt":string}
  T11 = enum16{"Config Save", "Config Load", "LastRUN Save", "LastRUN Load"}
  T12 = typedef "cmd_common.ctl" = enum16{"read", "write"}
  T13 = typedef "cmd_ini-RW.ctl" = enum16{"ini", "read", "write"}
  T14 = typedef "cmd_ini-add-read.ctl" = enum16{"ini", "add", "read"}
  T15 = typedef "GNSS-Ntrip ref.ctl" = cluster{"Mount point arr":refnum<vi>, "Select Mount points":refnum<vi>}
  T16 = enum8{"Enabled", "Disabled", "Disabled and Grayed Out"}
  T17 = typedef "GNSS-Ntrip config.ctl" = cluster{"Ntrip accounts":T10[], "Mount points":u16, "Ref r size":dbl, "TMarr limit":i32, "Sel NMEA type":enum16{"$GPGSV", "$GLGSV", "$GPGGA", "$GAGSV", "$GBGSV", "$GNGLL", "$GNGGA", "$GNGSA", "$GNRMC", "$GNVTG"}, "Local Time offset":u32, "GNSS Serial delay":u32, "Send Serial delay":u32, "Send Serial config":cluster{"NMEA out port":refnum<visa-resource-name>, "baud rate":u32}, "Mount point arr":string[]}
  T18 = cluster{"Gmap Lat":refnum<vi>, "Gmap Lon":refnum<vi>, "Lat Dbclk":refnum<vi>, "Lon Dbclk":refnum<vi>, "zoom":refnum<vi>, "PinDropMrkr":refnum<vi>}
  T19 = typedef "GNSS-Ntrip process val.ctl" = cluster{"GNSS time":string, "Ntrip conn":bool, "NMEA val":bool, "ycenter_TM":dbl, "xcenter_TM":dbl, "TM ref circles":cluster{"Y(E)":dbl, "X(N)":dbl}[], "RTCM recv-str":string, "GNSS Serail buff N":u32, "Sel NMEA type":enum16{"$GPGSV", "$GLGSV", "$GPGGA", "$GAGSV", "$GBGSV", "$GNGLL", "$GNGGA", "$GNGSA", "$GNRMC", "$GNVTG"}, "RTCM recv_sourcetable":string, "NMEA cluster":cluster{"GxGGA":string, "GxGSV":string, "GNRMC":string, "GxTXT":string, "GxGSA":string, "GxGLL":string}, "Sel NMEA str":string, "NMEA recv-str":string, "Ntrip Account DB index":u32, "Ntrip accounts DB":T10[]}
  T20 = typedef "gmap_fgv-cmd.ctl" = enum16{"marker type change", "save_image", "coll of points", "zoom n center markers", "add overlay reference", "read", "zoom", "set position by keyword", "set map provider", "map provider update", "create", "add marker", "clear marker", "close"}
  T21 = typedef "NMEA.lvlib/NMEA_LatitudeDirection.ctl" = enum16{"", "North", "South"}
  T22 = typedef "NMEA.lvlib/NMEA_LongitudeDirection.ctl" = enum16{"", "East", "West"}
  T23 = typedef "NMEA.lvlib/NMEA_GPS-Quality.ctl" = enum16{"Invalid", "GPS fix (SPS)", "DGPS fix", "PPS fix", "Real Time Kinematic", "Float RTK", "estimated", "Manual input mode", "Simulation mode"}
  T24 = cluster{"$GPGGA-message_OUT":cluster{"TimeStamp":timestamp, "Latitude":dbl, "Latitude-Direction":T21, "Longitude":dbl, "Longitude-Direction":T22, "GPS-Quality":T23, "N of Satellites":i32, "HDOP":dbl, "Altitude above Mean-Sea-Level":dbl, "Geoidal separation":dbl, "Time since last DGPS update":dbl, "DGPS reference station ID":i32}}
  T25 = cluster{"NA":u32, "valid":u32, "DGPS":u32, "RTK float":u32, "RTK fixed":u32}
  T26 = cluster{"TM array":cluster{"Y(E)":dbl, "X(N)":dbl}[]}
  T27 = cluster{"Ntrip tcp":bool, "GNSS serial":bool, "RTCM serial":bool, "Send serial":bool}
  T28 = cluster{"Ntrip accounts DB":T10[], "Select Mount points":u16, "Ref r size":dbl, "TMarr-size limit":i32, "Sel NMEA type":enum16{"$GPGSV", "$GLGSV", "$GPGGA", "$GAGSV", "$GBGSV", "$GNGLL", "$GNGGA", "$GNGSA", "$GNRMC", "$GNVTG"}, "Local Time offset":u32, "Send Serial delay ms":u32, "GNSS Serial delay":u32, "Send-Serial config":cluster{"NMEA out port":refnum<visa-resource-name>, "baud rate":u32}, "Mount point arr":string[]}
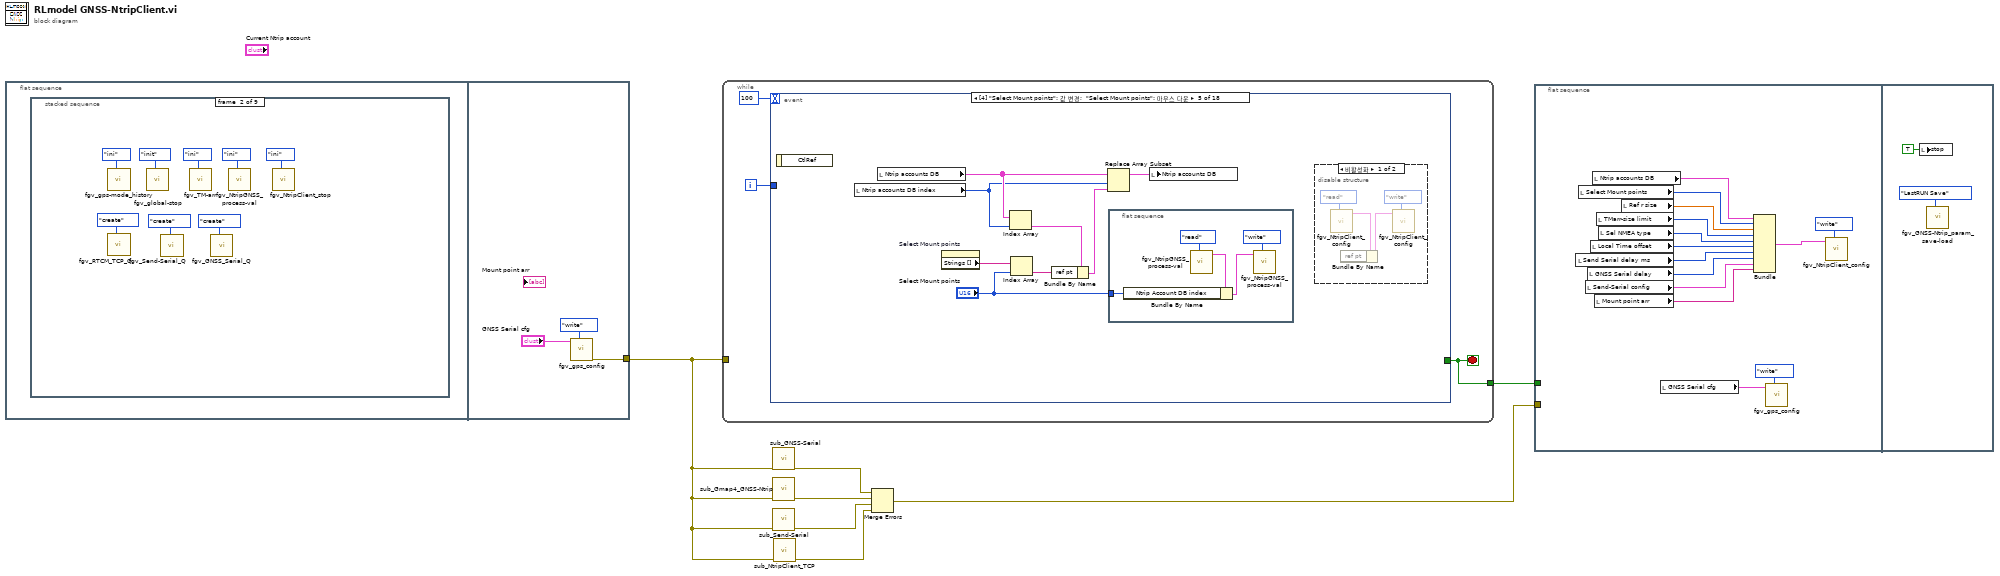
[diagram p0: block diagram]
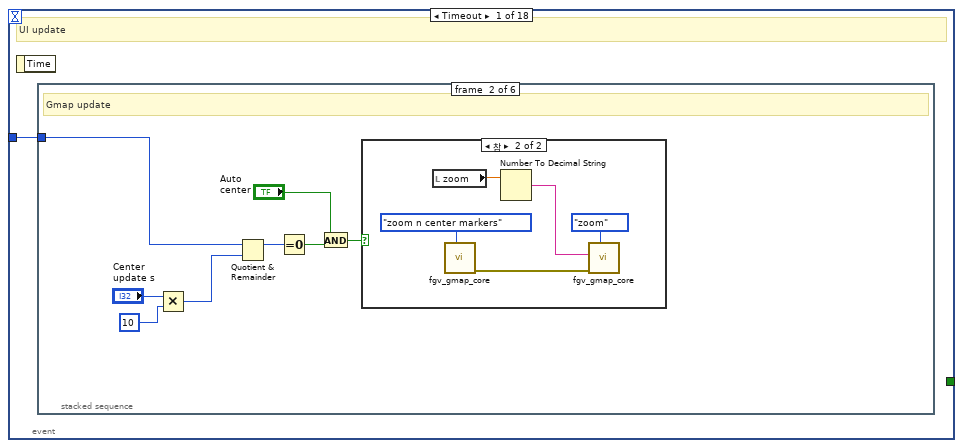
[diagram p2: hidden frame]
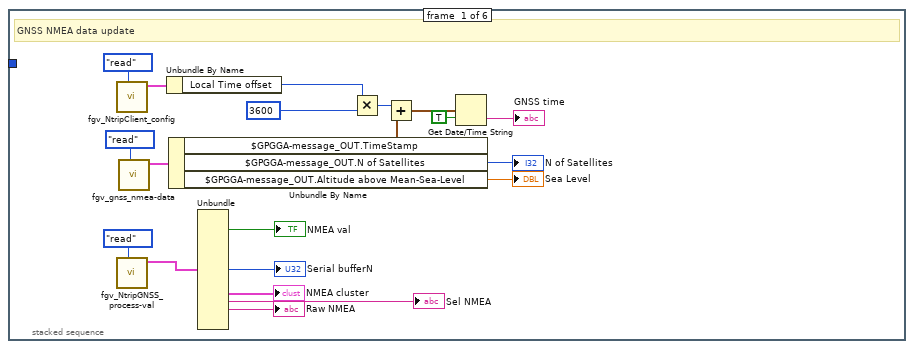
[diagram p3: hidden frame]
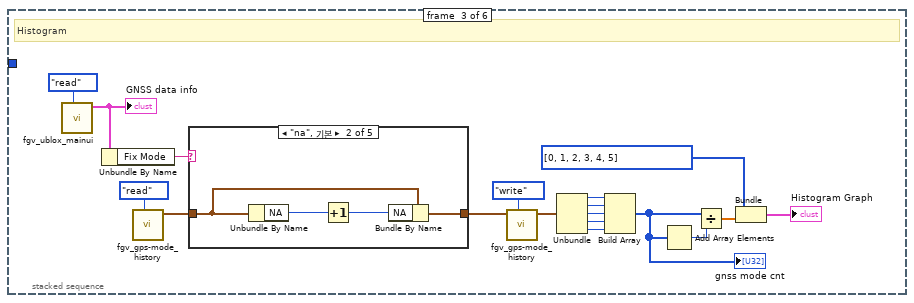
[diagram p5: hidden frame]
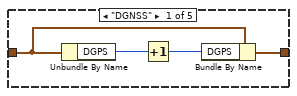
[diagram p6: hidden frame]
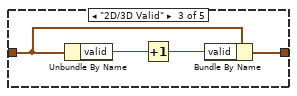
[diagram p7: hidden frame]
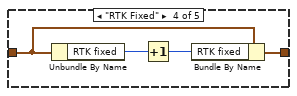
[diagram p8: hidden frame]
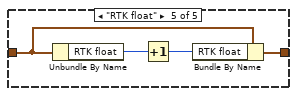
[diagram p9: hidden frame]
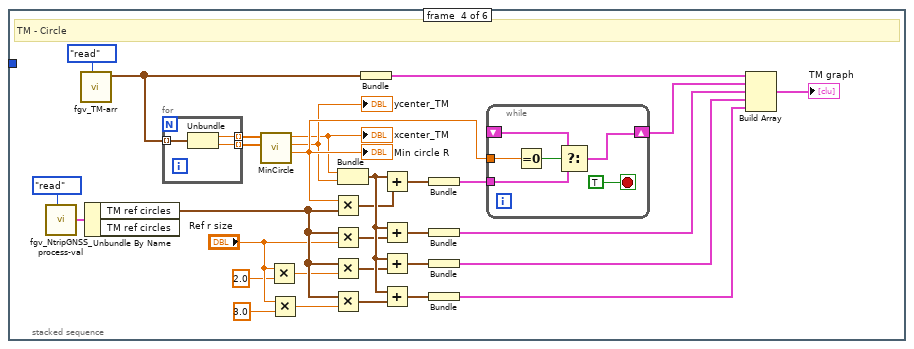
[diagram p10: hidden frame]
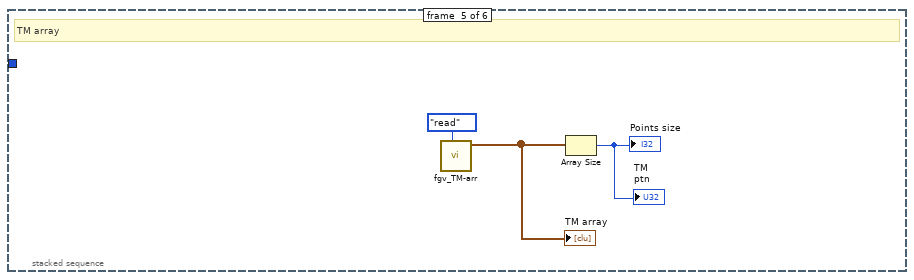
[diagram p11: hidden frame]
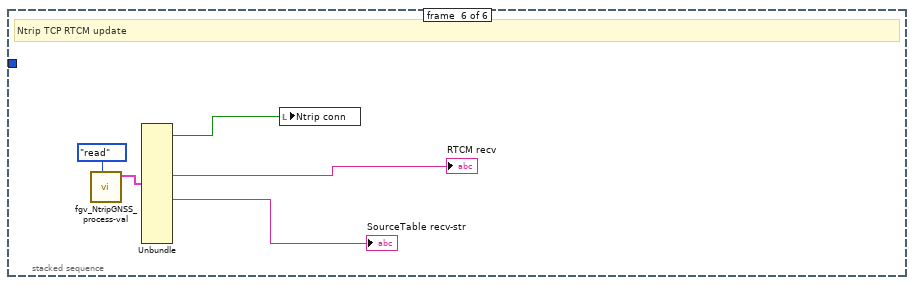
[diagram p12: hidden frame]
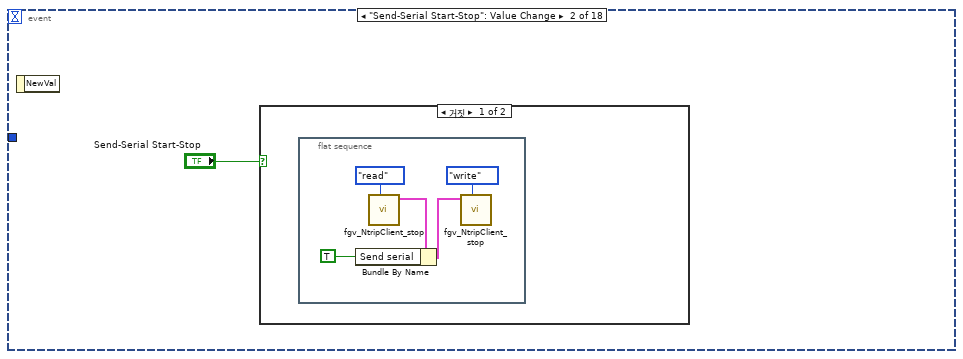
[diagram p13: hidden frame]
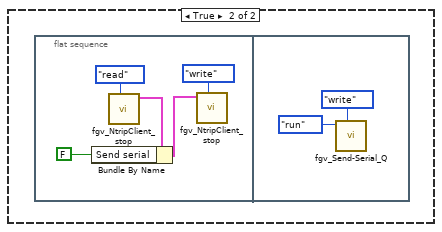
[diagram p14: hidden frame]
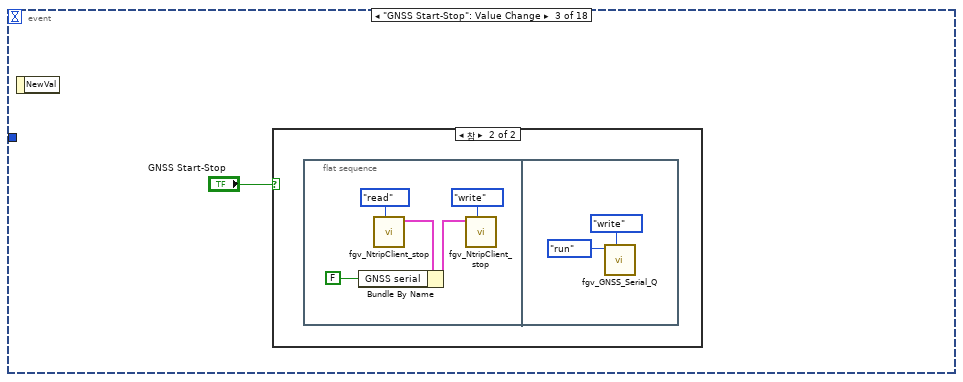
[diagram p15: hidden frame]
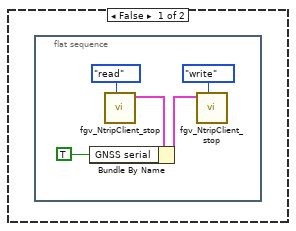
[diagram p16: hidden frame]
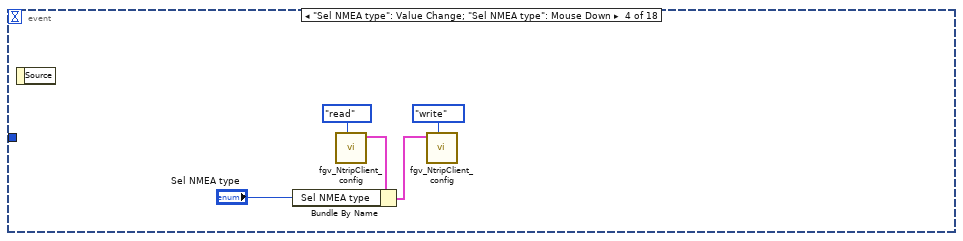
[diagram p17: hidden frame]
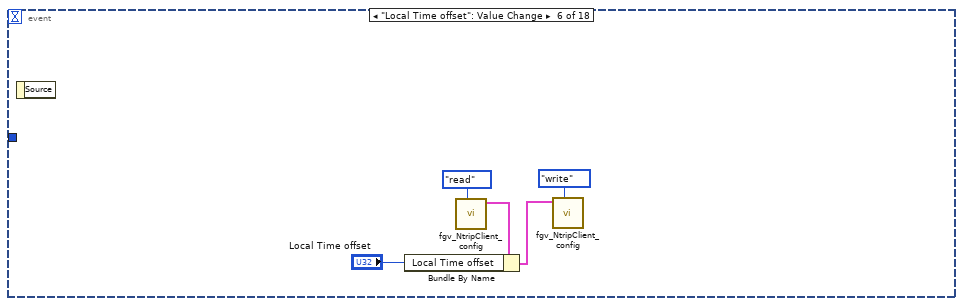
[diagram p19: hidden frame]
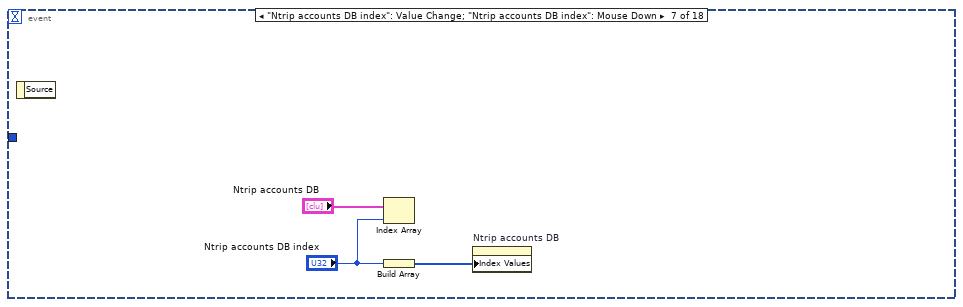
[diagram p20: hidden frame]
diagram:
  n1 = flat-sequence {
    tunnel: [w75] -> w6
    frame #0 {
      n2 = stacked-sequence {
        frame #0 {
          n3 = call "fgv_GNSS-Ntrip_param_save-load.vi"("ctl"=T11."LastRUN Load") -> ("error out"=w8:errorcluster)  [unwired: 9 in, 1 out]
          n4 = stacked-sequence {
            tunnel: w8 -> [_ _ _]
            frame #0 {
              n5 = call "fgv_gps_config.vi"("cmd"=enum16{"read", "write"}."read") -> ("GNSS cfg out"=w10:T8)  [unwired: 9 in, 1 out]
              n6 = local write "GNSS Serial cfg"(w10) -> ()
            }
            frame #1 {
              n7 = call "fgv_NtripClient_config.vi"("cmd"=cmd_common."read") -> ("config val out"=w22:T17)  [unwired: 10 in]
              n8 = Unbundle(w22) -> ("Ntrip accounts"=w20:T10[], "Mount points"=w19:u16, "Ref r size"=w18:dbl, "TMarr limit"=w17:i32, "Sel NMEA type"=w14:T7, "Local Time offset"=w13:u32, "GNSS Serial delay"=w12:u32, "Send Serial delay"=w21:u32, "Send Serial config"=w15:T9, "Mount point arr"=w16:string[])
              n9 = local write "Send Serial delay ms"(w21) -> ()
              n10 = local write "Select Mount points"(w19) -> ()
              n11 = local write "Ntrip accounts DB"(w20) -> ()
              n12 = local write "Send-Serial config"(w15) -> ()
              n13 = local write "GNSS Serial delay"(w12) -> ()
              n14 = local write "Local Time offset"(w13) -> ()
              n15 = local write "Mount point arr"(w16) -> ()
              n16 = local write "TMarr-size limit"(w17) -> ()
              n17 = property on="Select Mount points" class="Ring (엄격한)"("Strings []"=w16) -> ()  [unwired: 2 in, 2 out]
              n18 = local write "Sel NMEA type"(w14) -> ()
              n19 = local write "Ref r size"(w18) -> ()
            }
            frame #2 {
            }
          }
        }
        frame #1 {
          n20 = call "fgv_gps-mode_history.vi"("cmd"=cmd_ini-RW."ini") -> ()  [unwired: 10 in, 1 out]
          n21 = call "fgv_RTCM_TCP_Q.vi"("cmd"=enum16{"create", "write", "read", "close"}."create") -> ()  [unwired: 9 in, 2 out]
          n22 = call "fgv_global-stop.vi"("cmd"=enum16{"init", "stop", "read"}."init") -> ()  [unwired: 10 in, 1 out]
          n23 = call "fgv_Send-Serial_Q.vi"("cmd"=enum16{"create", "write", "read", "close"}."create") -> ()  [unwired: 9 in, 2 out]
          n24 = call "fgv_TM-arr.vi"("cmd"=cmd_ini-add-read."ini") -> ()  [unwired: 10 in, 1 out]
          n25 = call "fgv_GNSS_Serial_Q.vi"("cmd"=enum16{"create", "write", "read", "close"}."create") -> ()  [unwired: 9 in, 2 out]
          n26 = call "fgv_NtripGNSS_process-val.vi"("cmd"=cmd_ini-RW."ini") -> ()  [unwired: 10 in, 1 out]
          n27 = call "fgv_NtripClient_stop.vi"("cmd"=cmd_ini-RW."ini") -> ()  [unwired: 10 in, 1 out]
        }
        frame #2 {
          n28 = control-ref of="zoom"() -> (w43:refnum<vi>)
          n29 = control-ref of="Gmap Lat"() -> (w39:refnum<vi>)
          n30 = control-ref of="Gmap Lon"() -> (w40:refnum<vi>)
          n31 = control-ref of="Lat Dbclk"() -> (w41:refnum<vi>)
          n32 = control-ref of="Lon Dbclk"() -> (w42:refnum<vi>)
          n33 = control-ref of="PinDropMrkr"() -> (w44:refnum<vi>)
          n34 = control-ref of="Mount point arr"() -> (w36:refnum<vi>)
          n35 = control-ref of="Select Mount points"() -> (w33:refnum<vi>)
          n36 = Bundle("Gmap Lat"=w39, "Gmap Lon"=w40, "Lat Dbclk"=w41, "Lon Dbclk"=w42, "zoom"=w43, "PinDropMrkr"=w44) -> (w45:T18)  [unwired: 1 in]
          n37 = Bundle(cluster=T15 {"Mount point arr"=refnum, "Select Mount points"=refnum} ("ref 2"), "Mount point arr"=w36, "Select Mount points"=w33) -> (w34:T15)
          n38 = call "fgv_ctr-ref_gmap.vi"("cmd"=cmd_common."write", "ref in"=w45) -> ()  [unwired: 9 in, 1 out]
          n39 = call "fgv_ctrl-ref_cluster.vi"("cmd"=enum16{"read", "write"}."write", "ref"=w45) -> ()  [unwired: 9 in, 1 out]
          n40 = call "fgv_GNSS-Ntrip_ctrl-refs.vi"("cmd"=cmd_common."write", "ref"=w34) -> ()  [unwired: 9 in, 1 out]
        }
        frame #3 {
          n41 = call "fgv_NtripClient_config.vi"("cmd"=cmd_common."read") -> ("config val out"=w50:T17)  [unwired: 10 in]
          n42 = Bundle By Name(cluster=w50, "Send Serial config"="Send-Serial config") -> (w49:T17)
          n43 = call "fgv_NtripClient_config.vi"("cmd"=cmd_common."write", "config val"=w49) -> ()  [unwired: 9 in, 1 out]
        }
        frame #4 {
          n44 = call "sub_gmap_init.vi"("GMapControl"="GMapControl") -> ()  [unwired: 10 in, 1 out]
        }
        frame #5 {
          n45 = call "sub_log_fine-name.vi"() -> ("log path"=→"log path":string)  [unwired: 11 in]
        }
        frame #6 {
          w54 = 100
          n46 = Increment(x=w54) -> (x+1=w61:i32)
          n47 = Divide(x=6.283185307179586, y=w54) -> (x/y=w60:dbl)
          n48 = for {
            N: w61 -> [_]
            tunnel: w60 -> [w66]
            tunnel: [w62] -> w57 mode=indexing
            i -> [w67]
            n49 = Multiply(x=w66, y=w67) -> (x*y=w65:dbl)
            n50 = Sine & Cosine(0:w65) -> (1:w64:dbl, 2:w63:dbl)
            n51 = Bundle(w64, w63) -> (w62:cluster{dbl, dbl})  [unwired: 1 in]
          }
          n52 = call "fgv_NtripGNSS_process-val.vi"("cmd"=cmd_ini-RW."read") -> ("process val out"=w59:T19)  [unwired: 10 in]
          n53 = Bundle By Name(cluster=w59, "TM ref circles"=w57) -> (w58:T19)
          n54 = call "fgv_NtripGNSS_process-val.vi"("cmd"=cmd_ini-RW."write", "process val"=w58) -> ()  [unwired: 9 in, 1 out]
        }
        frame #7 {
          (unwired) "ICY 200 OK" ("정규식")
          w68 = "" ("read raw")
          w70 = FALSE ("정지")
          n55 = local write "Raw NMEA"(w68) -> ()
          n56 = local write "Sel NMEA"(w68) -> ()
          n57 = local write "RTCM recv"(w68) -> ()
          n58 = local write "SourceTable recv-str"(w68) -> ()
          n59 = local write "stop"(w70) -> ()
          n60 = local write "GNSS Start-Stop"(w70) -> ()
          n61 = local write "Send-Serial Start-Stop"(w70) -> ()
          n62 = local write "Ntrip connect"(w70) -> ()
          "Ntrip conn" <- FALSE ("ntrip val")
          "error out" <- errorcluster {"status"=FALSE, "code"=0, "source"=""} ("error out")
        }
        frame #8 {
          n63 = property on="TM\nptn" class="Slide (엄격한)"("Scale.Marker.Selection End"="TMarr-size limit") -> ()  [unwired: 2 in, 2 out]
          n64 = property on="Select Mount points" class="Ring (엄격한)"("DisabledEnum"=T16."Enabled" ("비활성화")) -> ()  [unwired: 2 in, 2 out]
        }
      }
    }
    frame #1 {
      n65 = call "fgv_gps_config.vi"("cmd"=enum16{"read", "write"}."write", "GNSS cfg"="GNSS Serial cfg") -> ("error out"=w75:errorcluster)  [unwired: 8 in, 1 out]
    }
  }
  n66 = while {
    tunnel: w6 -> [_]
    tunnel: [w79] -> w7
    i -> [w77]
    stop <- w79 stop-if-true
    n67 = event shown="[4] \"Select Mount points\": 값 변경;  \"Select Mount points\": 마우스 다운" {
      selector: _ -> [_ _ _ _ _ _ _ _ _ _ _ _ _ _ _ _ _ _]
      dyn-events: _ -> [_ _ _ _ _ _ _ _ _ _ _ _ _ _ _ _ _ _]
      timeout: 100 -> [_ _ _ _ _ _ _ _ _ _ _ _ _ _ _ _ _ _]
      tunnel: [_ _ _ _ _ _ _ _ _ w265 _ _ _ _ _ _ _ _] -> w79
      tunnel: w77 -> [w80 _ _ _ _ _ _ _ _ _ _ _ _ _ _ _ _ _]
      event Timeout {
        # "UI update"
        n68 = event-data() -> ()  [unwired: 1 in, 1 out]
        n69 = stacked-sequence {
          tunnel: w80 -> [_ w101 _ _ _ _]
          frame #0 {
            # "GNSS NMEA data update"
            n70 = call "fgv_NtripClient_config.vi"("cmd"=cmd_common."read") -> ("config val out"=w93:T17)  [unwired: 10 in]
            n71 = call "fgv_NtripGNSS_process-val.vi"("cmd"=cmd_ini-RW."read") -> ("process val out"=w86:T19)  [unwired: 10 in]
            n72 = call "fgv_gnss_nmea-data.vi"("cmd"=cmd_common."read") -> ("nmea-data out"=w98:T24)  [unwired: 10 in]
            n73 = Unbundle By Name(w93) -> ("Local Time offset"=w92:u32)
            n74 = Unbundle By Name(w98) -> ("$GPGGA-message_OUT.TimeStamp"=w97:timestamp, "$GPGGA-message_OUT.N of Satellites"=→"N of Satellites":i32, "$GPGGA-message_OUT.Altitude above Mean-Sea-Level"=→"Sea Level":dbl)
            n75 = Unbundle(w86) -> ("NMEA val"=→"NMEA val":bool, "GNSS Serail buff N"=→"Serial bufferN":u32, "NMEA cluster"=→"NMEA cluster":T6, "Sel NMEA str"=→"Sel NMEA":string, "NMEA recv-str"=→"Raw NMEA":string)  [unwired: 10 out]
            n76 = Multiply(x=w92, y=u32 3600) -> (x*y=w100:u32)
            n77 = Add(x=w100, y=w97) -> (x+y=w99:timestamp)
            n78 = Get Date/Time String(seconds (now)=w99, want seconds? (F)=TRUE ("초 보이기? (거짓)")) -> (time string=→"GNSS time":string)  [unwired: 1 in, 1 out]
          }
          frame #1 {
            # "Gmap update"
            n79 = Multiply(x="Center \nupdate s", y=10) -> (x*y=w102:i32)
            n80 = Quotient & Remainder(x=w101, y=w102) -> (x-y*floor(x/y)=w106:i32)  [unwired: 1 out]
            n81 = Equal To 0?(x=w106) -> (x = 0?=w107:bool)
            n82 = And(x="Auto\ncenter", y=w107) -> (x .and. y?=w108:bool)
            n83 = case shown="참" w108 {
              frame False {
              }
              frame True {
                n84 = local read "zoom"() -> (w113:dbl)
                n85 = call "fgv_gmap_core.vi"("cmd"=gmap_fgv-cmd."zoom n center markers") -> ("error out"=w109:errorcluster)  [unwired: 7 in, 3 out]
                n86 = Number To Decimal String(number=w113) -> (decimal integer string=w112:string)  [unwired: 1 in]
                n87 = call "fgv_gmap_core.vi"(7:"cmd"=gmap_fgv-cmd."zoom" ("cmd"), "error in"=w109, 10:"cmd"=w112) -> ()  [unwired: 5 in, 4 out]
              }
            }
          }
          frame #2 {
            # "Histogram"
            n88 = call "fgv_ublox_mainui.vi"("cmd"=cmd_common."read") -> ("MainUI gnss out"=w118:T3)  [unwired: 10 in]
            "GNSS data info" <- w118
            n89 = Unbundle By Name(w118) -> ("Fix Mode"=w119:string)
            n90 = call "fgv_gps-mode_history.vi"("cmd"=cmd_ini-RW."read") -> ("data out"=w120:T25)  [unwired: 10 in]
            n91 = case shown="\"na\", 기본" w119 {
              tunnel: w120 -> [w135 w139 w143 w147 w151]
              tunnel: [w134 w138 w142 w146 w150] -> w121
              frame "DGNSS" {
                n92 = Unbundle By Name(w135) -> ("DGPS"=w133:u32)
                n93 = Increment(x=w133) -> (x+1=w132:u32)
                n94 = Bundle By Name(cluster=w135, "DGPS"=w132) -> (w134:T25)
              }
              frame "na", Default {
                n95 = Unbundle By Name(w139) -> ("NA"=w137:u32)
                n96 = Increment(x=w137) -> (x+1=w136:u32)
                n97 = Bundle By Name(cluster=w139, "NA"=w136) -> (w138:T25)
              }
              frame "2D/3D Valid" {
                n98 = Unbundle By Name(w143) -> ("valid"=w141:u32)
                n99 = Increment(x=w141) -> (x+1=w140:u32)
                n100 = Bundle By Name(cluster=w143, "valid"=w140) -> (w142:T25)
              }
              frame "RTK Fixed" {
                n101 = Unbundle By Name(w147) -> ("RTK fixed"=w145:u32)
                n102 = Increment(x=w145) -> (x+1=w144:u32)
                n103 = Bundle By Name(cluster=w147, "RTK fixed"=w144) -> (w146:T25)
              }
              frame "RTK float" {
                n104 = Unbundle By Name(w151) -> ("RTK float"=w149:u32)
                n105 = Increment(x=w149) -> (x+1=w148:u32)
                n106 = Bundle By Name(cluster=w151, "RTK float"=w148) -> (w150:T25)
              }
            }
            n107 = call "fgv_gps-mode_history.vi"("cmd"=cmd_ini-RW."write", "data"=w121) -> ("data out"=w122:T25)  [unwired: 9 in]
            n108 = Unbundle(w122) -> ("NA"=w123:u32, "valid"=w127:u32, "DGPS"=w126:u32, "RTK float"=w125:u32, "RTK fixed"=w124:u32)
            n109 = Build Array(w123, w127, w126, w125, w124) -> (w131:u32[])
            "gnss mode cnt" <- w131
            n110 = Add Array Elements(numeric array=w131) -> (sum=w129:u32)
            n111 = Divide(x=w131, y=w129) -> (x/y=w130:dbl[])
            n112 = Bundle(i32[] [0, 1, 2, 3, 4, 5], w130) -> (→"Histogram Graph":cluster{i32[], dbl[]})  [unwired: 1 in]
          }
          frame #3 {
            # "TM - Circle"
            n113 = call "fgv_NtripGNSS_process-val.vi"("cmd"=cmd_ini-RW."read") -> ("process val out"=w180:T19)  [unwired: 10 in]
            n114 = call "fgv_TM-arr.vi"("cmd"=cmd_ini-add-read."read") -> ("TM array"=w182:cluster{"Y(E)":dbl, "X(N)":dbl}[])  [unwired: 10 in]
            n115 = Unbundle By Name(w180) -> ("TM ref circles"=w181:cluster{"Y(E)":dbl, "X(N)":dbl}[])  [unwired: 1 out]
            n116 = for {
              tunnel: [w191] -> w157 mode=indexing
              tunnel: [w190] -> w158 mode=indexing
              tunnel: w182 -> [w189] mode=indexing
              n117 = Unbundle(w189) -> ("Y(E)"=w191:dbl, "X(N)"=w190:dbl)
            }
            n118 = call "MinCircle.vi"("y"=w158, "x"=w157) -> ("r"=w167:dbl, "yc"=w160:dbl, "xc"=w159:dbl)  [unwired: 6 in, 1 out]
            "xcenter_TM" <- w159
            "ycenter_TM" <- w160
            "Min circle R" <- w167
            n119 = Multiply(x="Ref r size", y=2.0) -> (x*y=w172:dbl)
            n120 = Multiply(x="Ref r size", y=3.0) -> (x*y=w153:dbl)
            n121 = Multiply(x=w167, y=w181) -> (x*y=w161:cluster{"Y(E)":dbl, "X(N)":dbl}[])
            n122 = Multiply(x=w181, y="Ref r size") -> (x*y=w171:cluster{"Y(E)":dbl, "X(N)":dbl}[])
            n123 = Multiply(x=w181, y=w172) -> (x*y=w170:cluster{"Y(E)":dbl, "X(N)":dbl}[])
            n124 = Multiply(x=w181, y=w153) -> (x*y=w173:cluster{"Y(E)":dbl, "X(N)":dbl}[])
            n125 = Bundle("xc"=w159, "yc"=w160) -> (w174:cluster{"xc":dbl, "yc":dbl})  [unwired: 1 in]
            n126 = Bundle("TM array"=w182) -> (w163:T26)  [unwired: 1 in]
            n127 = Add(x=w174, y=w161) -> (x+y=w162:cluster{dbl, dbl}[])
            n128 = Add(x=w174, y=w171) -> (x+y=w168:cluster{dbl, dbl}[])
            n129 = Add(x=w174, y=w170) -> (x+y=w176:cluster{dbl, dbl}[])
            n130 = Add(x=w174, y=w173) -> (x+y=w175:cluster{dbl, dbl}[])
            n131 = Bundle(w162) -> (w165:cluster{cluster{dbl, dbl}[]})  [unwired: 1 in]
            n132 = Bundle(w168) -> (w169:cluster{cluster{dbl, dbl}[]})  [unwired: 1 in]
            n133 = Bundle(w176) -> (w177:cluster{cluster{dbl, dbl}[]})  [unwired: 1 in]
            n134 = Bundle(w175) -> (w178:cluster{cluster{dbl, dbl}[]})  [unwired: 1 in]
            n135 = while {
              shift-right: [w183] -> w166
              shift-left: _ -> [w185]
              tunnel: w167 -> [w187]
              tunnel: w165 -> [w184]
              stop <- TRUE stop-if-true
              n136 = Equal To 0?(x=w187) -> (x = 0?=w186:bool)
              n137 = Select(t=w185, s=w186, f=w184) -> (s? t:f=w183:cluster{cluster{dbl, dbl}[]})
            }
            n138 = Build Array(w163, w166, w169, w177, w178) -> (→"TM graph":T2)
          }
          frame #4 {
            # "TM array"
            n139 = call "fgv_TM-arr.vi"("cmd"=cmd_ini-add-read."read") -> ("TM array"=w192:cluster{"Y(E)":dbl, "X(N)":dbl}[])  [unwired: 10 in]
            "TM array" <- w192
            n140 = Array Size(array=w192) -> (size(s)=→"Points size" →"TM\nptn":i32)
          }
          frame #5 {
            # "Ntrip TCP RTCM update"
            n141 = call "fgv_NtripGNSS_process-val.vi"("cmd"=cmd_ini-RW."read") -> ("process val out"=w198:T19)  [unwired: 10 in]
            n142 = Unbundle(w198) -> ("Ntrip conn"=w195:bool, "RTCM recv-str"=→"RTCM recv":string, "RTCM recv_sourcetable"=→"SourceTable recv-str":string)  [unwired: 12 out]
            n143 = local write "Ntrip conn"(w195) -> ()
          }
        }
      }
      event "Send-Serial Start-Stop": Value Change {
        n144 = event-data() -> ()  [unwired: 1 in, 1 out]
        n145 = case shown="거짓" "Send-Serial Start-Stop" {
          frame False {
            n146 = flat-sequence {
              frame #0 {
                n147 = call "fgv_NtripClient_stop.vi"("cmd"=cmd_ini-RW."read") -> ("local stops out"=w203:T27)  [unwired: 10 in]
                n148 = Bundle By Name(cluster=w203, "Send serial"=TRUE ("Ntrip tcp")) -> (w202:T27)
                n149 = call "fgv_NtripClient_stop.vi"("cmd"=cmd_ini-RW."write", "local stops"=w202) -> ()  [unwired: 9 in, 1 out]
              }
            }
          }
          frame True {
            n150 = flat-sequence {
              frame #0 {
                n151 = call "fgv_NtripClient_stop.vi"("cmd"=cmd_ini-RW."read") -> ("local stops out"=w208:T27)  [unwired: 10 in]
                n152 = Bundle By Name(cluster=w208, "Send serial"=FALSE ("Ntrip tcp")) -> (w207:T27)
                n153 = call "fgv_NtripClient_stop.vi"("cmd"=cmd_ini-RW."write", "local stops"=w207) -> ()  [unwired: 9 in, 1 out]
              }
              frame #1 {
                n154 = call "fgv_Send-Serial_Q.vi"("cmd"=enum16{"create", "write", "read", "close"}."write", "data"=enum16{"run", "check", "stop"}."run") -> ()  [unwired: 8 in, 2 out]
              }
            }
          }
        }
      }
      event "GNSS Start-Stop": Value Change {
        n155 = event-data() -> ()  [unwired: 1 in, 1 out]
        n156 = case shown="참" "GNSS Start-Stop" {
          frame False {
            n157 = flat-sequence {
              frame #0 {
                n158 = call "fgv_NtripClient_stop.vi"("cmd"=cmd_ini-RW."read") -> ("local stops out"=w216:T27)  [unwired: 10 in]
                n159 = Bundle By Name(cluster=w216, "GNSS serial"=TRUE ("Ntrip tcp")) -> (w215:T27)
                n160 = call "fgv_NtripClient_stop.vi"("cmd"=cmd_ini-RW."write", "local stops"=w215) -> ()  [unwired: 9 in, 1 out]
              }
            }
          }
          frame True {
            n161 = flat-sequence {
              frame #0 {
                n162 = call "fgv_NtripClient_stop.vi"("cmd"=cmd_ini-RW."read") -> ("local stops out"=w221:T27)  [unwired: 10 in]
                n163 = Bundle By Name(cluster=w221, "GNSS serial"=FALSE ("Ntrip tcp")) -> (w220:T27)
                n164 = call "fgv_NtripClient_stop.vi"("cmd"=cmd_ini-RW."write", "local stops"=w220) -> ()  [unwired: 9 in, 1 out]
              }
              frame #1 {
                n165 = call "fgv_GNSS_Serial_Q.vi"("cmd"=enum16{"create", "write", "read", "close"}."write", "data"=enum16{"run", "check", "stop"}."run") -> ()  [unwired: 8 in, 2 out]
              }
            }
          }
        }
      }
      event "Sel NMEA type": Value Change; "Sel NMEA type": Mouse Down {
        n166 = event-data() -> ()  [unwired: 1 in, 1 out]
        n167 = call "fgv_NtripClient_config.vi"("cmd"=cmd_common."read") -> ("config val out"=w230:T17)  [unwired: 10 in]
        n168 = Bundle By Name(cluster=w230, "Sel NMEA type"="Sel NMEA type") -> (w229:T17)
        n169 = call "fgv_NtripClient_config.vi"("cmd"=cmd_common."write", "config val"=w229) -> ()  [unwired: 9 in, 1 out]
      }
      event "Select Mount points": Value Change; "Select Mount points": Mouse Down {
        n170 = event-data() -> ()  [unwired: 1 in, 1 out]
        n171 = local read "Ntrip accounts DB index"() -> (w236:u32)
        n172 = local read "Ntrip accounts DB"() -> (w237:T10[])
        n173 = property on="Select Mount points" class="Ring (엄격한)"() -> ("Strings []"=w238:string[])  [unwired: 2 in, 2 out]
        n174 = Index Array(array=w237, index=w236) -> (element=w235:T10)
        n175 = Index Array(array=w238, index="Select Mount points") -> (element=w234:string)
        n176 = Bundle By Name(cluster=w235, "ref pt"=w234) -> (w233:T10)
        n177 = Replace Array Subset(array=w237, new element=w233, index=w236) -> (w232:T10[])
        n178 = flat-sequence {
          tunnel: "Select Mount points" -> [w240]
          frame #0 {
            n179 = call "fgv_NtripGNSS_process-val.vi"("cmd"=cmd_ini-RW."read") -> ("process val out"=w241:T19)  [unwired: 10 in]
            n180 = Bundle By Name(cluster=w241, "Ntrip Account DB index"=w240) -> (w239:T19)
            n181 = call "fgv_NtripGNSS_process-val.vi"("cmd"=cmd_ini-RW."write", "process val"=w239) -> ()  [unwired: 9 in, 1 out]
          }
        }
        n182 = local write "Ntrip accounts DB"(w232) -> ()
        n183 = disable-structure shown="비활성화" {
          frame Disabled {
            n184 = call "fgv_NtripClient_config.vi"("cmd"=cmd_common."read") -> ("config val out"=w247:T17)  [unwired: 10 in]
            n185 = Bundle By Name(cluster=w247) -> (w246:T17)  [unwired: 1 in]
            n186 = call "fgv_NtripClient_config.vi"("cmd"=cmd_common."write", "config val"=w246) -> ()  [unwired: 9 in, 1 out]
          }
          frame Enabled {
          }
        }
      }
      event "Local Time offset": Value Change {
        n187 = event-data() -> ()  [unwired: 1 in, 1 out]
        n188 = call "fgv_NtripClient_config.vi"("cmd"=cmd_common."read") -> ("config val out"=w250:T17)  [unwired: 10 in]
        n189 = Bundle By Name(cluster=w250, "Local Time offset"="Local Time offset") -> (w248:T17)
        n190 = call "fgv_NtripClient_config.vi"("cmd"=cmd_common."write", "config val"=w248) -> ()  [unwired: 9 in, 1 out]
      }
      event "Ntrip accounts DB index": Value Change; "Ntrip accounts DB index": Mouse Down {
        n191 = event-data() -> ()  [unwired: 1 in, 1 out]
        n192 = Index Array(array="Ntrip accounts DB", index="Ntrip accounts DB index") -> ()  [unwired: 1 out]
        n193 = Build Array("Ntrip accounts DB index") -> (w253:u32[])
        n194 = property on="Ntrip accounts DB" class="Arr (엄격한)"("Index Values"=w253) -> ()  [unwired: 2 in, 2 out]
      }
      event "GNSS Serial delay": Value Change {
        n195 = event-data() -> ()  [unwired: 1 in, 1 out]
        n196 = call "fgv_NtripClient_config.vi"("cmd"=cmd_common."read") -> ("config val out"=w258:T17)  [unwired: 10 in]
        n197 = Bundle By Name(cluster=w258, "GNSS Serial delay"="GNSS Serial delay") -> (w257:T17)
        n198 = call "fgv_NtripClient_config.vi"("cmd"=cmd_common."write", "config val"=w257) -> ()  [unwired: 9 in, 1 out]
      }
      event "TMarr-size limit": Value Change {
        n199 = event-data() -> ()  [unwired: 1 in, 1 out]
        n200 = local read "TMarr-size limit"() -> (w261:i32)
        n201 = property on="TM\nptn" class="Slide (엄격한)"("Scale.Marker.Selection End"=w261) -> ()  [unwired: 2 in, 2 out]
      }
      event "stop": Value Change {
        n202 = event-data() -> ()  [unwired: 1 in, 1 out]
        n203 = call "fgv_GNSS_Serial_Q.vi"("cmd"=enum16{"create", "write", "read", "close"}."close") -> ()  [unwired: 9 in, 2 out]
        n204 = call "fgv_RTCM_TCP_Q.vi"("cmd"=enum16{"create", "write", "read", "close"}."close") -> ()  [unwired: 9 in, 2 out]
        n205 = call "fgv_Send-Serial_Q.vi"("cmd"=enum16{"create", "write", "read", "close"}."close") -> ()  [unwired: 9 in, 2 out]
        n206 = call "fgv_global-stop.vi"("cmd"=enum16{"init", "stop", "read"}."stop") -> ("val_out"=w265:bool)  [unwired: 10 in]
      }
      event "update mount point": Value Change {
        n207 = event-data() -> ()  [unwired: 1 in, 1 out]
        n208 = call "fgv_RTCM_TCP_Q.vi"("cmd"=enum16{"create", "write", "read", "close"}."write", "data"=enum16{"run", "check", "stop"}."check") -> ()  [unwired: 8 in, 2 out]
      }
      event "Ntrip accounts DB": Value Change {
        n209 = event-data() -> ()  [unwired: 1 in, 1 out]
      }
      event "gmap center": Value Change {
        n210 = event-data() -> ()  [unwired: 1 in, 1 out]
        n211 = call "fgv_gmap_core.vi"("cmd"=gmap_fgv-cmd."zoom n center markers") -> ("error out"=w269:errorcluster)  [unwired: 7 in, 3 out]
        n212 = local read "zoom"() -> (w272:dbl)
        n213 = Number To Decimal String(number=w272) -> (decimal integer string=w271:string)  [unwired: 1 in]
        n214 = call "fgv_gmap_core.vi"(7:"cmd"=gmap_fgv-cmd."zoom" ("cmd"), "error in"=w269, 10:"cmd"=w271) -> ()  [unwired: 5 in, 4 out]
      }
      event "Ntrip connect": Value Change {
        n215 = event-data() -> ()  [unwired: 1 in, 1 out]
        n216 = case shown="참" "Ntrip connect" {
          frame False {
            n217 = call "fgv_NtripClient_stop.vi"("cmd"=cmd_ini-RW."read") -> ("local stops out"=w277:T27)  [unwired: 10 in]
            n218 = Bundle By Name(cluster=w277, "Ntrip tcp"=TRUE) -> (w276:T27)
            n219 = call "fgv_NtripClient_stop.vi"("cmd"=cmd_ini-RW."write", "local stops"=w276) -> ()  [unwired: 9 in, 1 out]
          }
          frame True {
            n220 = flat-sequence {
              frame #0 {
                n221 = call "fgv_NtripClient_stop.vi"("cmd"=cmd_ini-RW."read") -> ("local stops out"=w284:T27)  [unwired: 10 in]
                n222 = Bundle By Name(cluster=w284, "Ntrip tcp"=FALSE) -> (w283:T27)
                n223 = call "fgv_NtripClient_stop.vi"("cmd"=cmd_ini-RW."write", "local stops"=w283) -> ()  [unwired: 9 in, 1 out]
              }
              frame #1 {
                n224 = call "fgv_RTCM_TCP_Q.vi"("cmd"=enum16{"create", "write", "read", "close"}."write", "data"=enum16{"run", "check", "stop"}."run") -> ()  [unwired: 8 in, 2 out]
              }
            }
          }
        }
      }
      event "tm data reset": Value Change {
        # "TM GPS data array reset"
        n225 = event-data() -> ()  [unwired: 1 in, 1 out]
        n226 = case shown="참" "tm data reset" {
          frame False {
          }
          frame True {
            n227 = call "fgv_TM-arr.vi"("cmd"=cmd_ini-add-read."ini") -> ()  [unwired: 10 in, 1 out]
          }
        }
      }
      event "zoom": Value Change {
        n228 = event-data() -> ()  [unwired: 1 in, 1 out]
        n229 = local read "zoom"() -> (w290:dbl)
        n230 = Number To Decimal String(number=w290) -> (decimal integer string=w289:string)  [unwired: 1 in]
        n231 = call "fgv_gmap_core.vi"(7:"cmd"=gmap_fgv-cmd."zoom" ("cmd"), 10:"cmd"=w289) -> ()  [unwired: 6 in, 4 out]
      }
      event "gnss mode check": Value Change {
        n232 = event-data() -> ()  [unwired: 1 in, 1 out]
        n233 = call "fgv_gps-mode_history.vi"("cmd"=cmd_ini-RW."ini") -> ()  [unwired: 10 in, 1 out]
      }
      event Value Change {
        n234 = event-data() -> ()  [unwired: 1 in, 1 out]
        n235 = local read "GNSS Serial cfg"() -> (w293:T8)
        n236 = call "fgv_gps_config.vi"("cmd"=enum16{"read", "write"}."write", "GNSS cfg"=w293) -> ()  [unwired: 8 in, 2 out]
      }
    }
  }
  n237 = call "sub_GNSS-Serial.vi"("error in"=w6) -> ("error out"=w2:errorcluster)  [unwired: 10 in]
  n238 = call "sub_Gmap4_GNSS-Ntrip.vi"("error in"=w6) -> ("error out"=w3:errorcluster)  [unwired: 10 in]
  n239 = call "sub_Send-Serial.vi"("error in"=w6) -> ("error out"=w4:errorcluster)  [unwired: 10 in]
  n240 = call "sub_NtripClient_TCP.vi"("error in"=w6) -> ("error out"=w5:errorcluster)  [unwired: 10 in]
  n241 = Merge Errors(w2, w3, w4, w5) -> (w1:errorcluster)
  n242 = flat-sequence {
    tunnel: w7 -> [_]
    tunnel: w1 -> [_]
    frame #0 {
      n243 = local read "Send Serial delay ms"() -> (w297:u32)
      n244 = local read "Select Mount points"() -> (w304:u16)
      n245 = local read "Send-Serial config"() -> (w299:T9)
      n246 = local read "GNSS Serial delay"() -> (w298:u32)
      n247 = local read "Local Time offset"() -> (w296:u32)
      n248 = local read "Ntrip accounts DB"() -> (w305:T10[])
      n249 = local read "Mount point arr"() -> (w300:string[])
      n250 = local read "TMarr-size limit"() -> (w302:i32)
      n251 = local read "Sel NMEA type"() -> (w301:T7)
      n252 = local read "Ref r size"() -> (w303:dbl)
      n253 = local read "GNSS Serial cfg"() -> (w306:T8)
      n254 = Bundle("Ntrip accounts DB"=w305, "Select Mount points"=w304, "Ref r size"=w303, "TMarr-size limit"=w302, "Sel NMEA type"=w301, "Local Time offset"=w296, "Send Serial delay ms"=w297, "GNSS Serial delay"=w298, "Send-Serial config"=w299, "Mount point arr"=w300) -> (w295:T28)  [unwired: 1 in]
      n255 = call "fgv_gps_config.vi"("cmd"=enum16{"read", "write"}."write", "GNSS cfg"=w306) -> ()  [unwired: 8 in, 2 out]
      n256 = call "fgv_NtripClient_config.vi"("cmd"=cmd_common."write", "config val"=w295) -> ()  [unwired: 9 in, 1 out]
    }
    frame #1 {
      n257 = local write "stop"(TRUE ("stop")) -> ()
      n258 = call "fgv_GNSS-Ntrip_param_save-load.vi"("ctl"=T11."LastRUN Save") -> ()  [unwired: 9 in, 2 out]
    }
  }
